vi "UHR-Fleezers Control (fpga) - avogadro 1.vi"() -> ()   [LabVIEW 2014]
doc: "UHR-Fleezers Instrument Control Code (fpga)"
uses:
  <vilib>/Platform/TimedLoop/XDataNode/timing_clust.ctl
  <vilib>/Platform/TimedLoop/XDataNode/nitl_modes.ctl
  <vilib>/Platform/TimedLoop/XDataNode/wakeup.ctl
  <vilib>/rvi/Emulation/niFpgaGetClockAttributes.vi
  <vilib>/rvi/Emulation/niFpgaSctlEmulationGetInTimedLoop.vi
  <vilib>/rvi/Emulation/niFpgaEmulationReportErrorSimple.vi
  <vilib>/rvi/Emulation/niFpgaProcessEmulError.vi
  <vilib>/rvi/eio/common/nirviEmuTemplateMethod_errors.vi
  <vilib>/rvi/interface/RandomDataEmulation/niFpgaRandomDataHandleErrors.vi
  <vilib>/rvi/Emulation/niFpgaCriticalErrorInLSC.vi
  <vilib>/eio/EIONode/EIONode.xnode
  <vilib>/eio/EIOMethodNode/EIOMethodNode.xnode
  <vilib>/rvi/DataTransferAndStorage/Container/XNode/niFpgaContainer.xnode
  <vilib>/rvi/interface/RandomDataEmulation/nirviRandomDataFpgaReadWriteTemplate.vi
  <vilib>/addons/control/pid/fpga.llb/XNode/niFpgaPID.xnode
  <vilib>/Platform/TimedLoop/XDataNode/XDataNode.xnode
  <vilib>/Platform/TimedLoop/XDataNode/XDNodeRunTimeDep.lvlib
panel:
  in  "Tab Control":T1(tab)=enum."MCL trap control"
  in  "Set 3":bool
  in  "Set 2":bool=TRUE
  in  "Set 1":bool=TRUE
  in  "Trap Pos to FIFO":bool
  in  "N of AI1 Int Acq Sets":i16=2 min=1 max=3 step=1
  out "AI Late Counter":u8
  in  "ai count":u16=400
  in  "+ phase":bool
  in  "Phase count adjustment":i16
  out "Relative phase":i16
  in  "AI to FIFO":bool
  out "BD1 Frequency Out 1":u64
  out "BD1 Frequency Out 2":u64
  out "Trap Pos FIFO Timeout":u16
  out "Trap AI FIFO Timeout":u16
  in  "Trap FIFO Set Timeout":i32
  in  "Tab Control 2":T2(tab)
  in  "FB output range":cluster{"output low":i16, "output high":i16}={"output low"=0, "output high"=3000}
  in  "FB Gains":T3={"proportional gain (Kc)"=10, "integral gain (Kc*Ts/Ti)"=5, "derivative gain (Kc*Td/Ts)"=0}
  in  "RD":bool
  in  "Swap F1 and F2":bool
  in  "Cont. Scan":bool
  in  "Abort scan":bool
  in  "Cycles per step":u64
  in  "Scan BD":bool
  in  "Number of scans":u16
  in  "Scan steps":u64
  in  "Scan freq.  increment":i64
  out "Scanning":bool
  in  "Start scan":bool
  in  "OSK Bd 1":bool
  in  "Reset Bd 1":bool
  in  "PMODE":bool
  in  "Direct RF Box \nCommunication":bool
  in  "Data BD 2":u8 format="%08b"
  in  "Data BD 1":u8 format="%08b"
  in  "Address":u8 format="%02x"
  in  "Update Data":bool
  in  "FPGA Controls\n RF Box":bool
  in  "Number Interlace Cycles":u8=2 min=1 max=3
  in  "Interlace Off Parameters":u8=1 min=1 max=3
  in  "Interlace ON/OFF":bool
  out "DIO Relative phase":i16
  in  "Phase count adjustment (DIO)":i16
  in  "+ phase (DIO)":bool
  out "DIO Late Counter":u8
  in  "DIO count 1 (ticks)":u16=400
  in  "DIO count 2 (ticks)":u16=400
  in  "DIO count 3 (ticks)":u16=400
  out "AI2 Y Sum Set 2":i16
  out "AI2 Y Sum Set 1":i16
  in  "FB Setpoint Set 1":i16 min=0 step=1
  in  "FB Reset Set 1":bool
  in  "FB On/Off Set 1":bool
  in  "FB Reset Set 2":bool
  in  "FB On/Off Set 2":bool
  in  "FB Setpoint Set 2":i16 min=0 step=1
  out "Scan I":u64
  in  "Amp switch delay":u8=5
  in  "BD 2 Amplitude 1":u16
  in  "BD 1 Amplitude 1":u16
  in  "BD 2 Frequency 1":u64
  in  "BD 1 Frequency 1":u64
  in  "BD 2 Amplitude 2":u16
  in  "BD 1 Amplitude 2":u16
  in  "BD 2 Frequency 2":u64
  in  "BD 1 Frequency 2":u64
  in  "BD 2 Amplitude 3":u16
  in  "BD 1 Amplitude 3":u16
  in  "BD 2 Frequency 3":u64
  in  "BD 1 Frequency 3":u64
  in  "BD 1 Delay (ticks)":u8
  in  "BD 2 Delay (Ticks)":u8 caption="Count(Ticks)"
  in  "Next trap write delay (ticks)":u8 caption="Count(Ticks)"
  out "Piezo X out":i16
  out "Piezo Y out":i16
  in  "Piezo Trap ON/Off (AO3)":i16
  in  "Piezo Trap X (AO5)":i16
  in  "Piezo Trap Y (AO4)":i16
  in  "Trap pos. FB Range":T4={"FB2 output low"=-1.0, "FB2 output high"=0.999969482421875}
  in  "FB Min frequency":u64
  in  "FB Max Frequency":u64
  in  "Dynamic Force FB (Ronen)":bool
  in  "Negate Diff?":bool
  in  "Diff FB Measurement?":bool
  in  "FB Trig Integrate":u32=1
  out "TTrig?":bool
  in  "TTrig Negate Pos":bool=TRUE
  out "Trap Pos FB Int Signal":fxp<+/-,24,9> format="%.18g"
  out "Trap Pos FB Int-Norm Signal":fxp<+/-,16,1> format="%.16g"
  in  "FPGA TTrig Thresh":i64
  in  "FPGA Trap Trig":bool
  out "Trap Pos FB Action":i64
  in  "Trap Pos. FB Offset Factor":i64
  in  "Trap Pos. FB Mult Factor":i64=2
  in  "Trap Pos. FB Reset":bool
  in  "Trap Pos FB Monitor T1 or T2":bool
  in  "AI1 X Scale":u16
  in  "Trap Pos FB Int Count":u16=100
  in  "Trap Pos FB Negate Action":bool
  out "AI1 X Set 2":fxp<+/-,16,1>
  out "AI1 X Set 1":fxp<+/-,16,1>
  in  "Trap Pos. FB SP":fxp<+/-,16,1>
  in  "Force feedback":bool
  out "TTrig Sig":i64
  out "TTrig Fin Thresh":i64
  in  "B factor":fxp<+/-,32,16>
  in  "Trap Pos. FB Gains":T5={"proportional gain (Kc)"=0.999969482421875, "integral gain (Kc*Ts/Ti)"=0.999969482421875, "derivative gain (Kc*Td/Ts)"=0.0}
  in  "ScanTrap 3 or Fl-laser":bool
  in  "1D or 2D Scan?":bool
  in  "Abort scan (MCL)":bool
  in  "MCL Scan Axis":bool
  in  "Cont. Scan (MCL)":bool
  out "Scan I (MCL)":u64
  in  "Number of scans (MCL)":u16
  out "Scanning MCL":bool
  in  "Scan steps (MCL)":u64
  in  "Cycles per step (MCL)":u64
  in  "Scan freq.  increment (MCL)":i16
  in  "Start scan (MCL)":bool
  in  "AO2 (X)":i16
  in  "AO1 (Y)":i16
  out "MCL Late Counter":u8
  in  "MCL count":u32=800
  out "MCL Relative Phase":i16
  in  "Phase count adjustment (MCL)":i16
  in  "+ phase (MCL)":bool
  out "APD2 int gate":bool
  out "APD3 out state":bool
  in  "APD Gate Operating Mode":u8 max=2 step=1
  in  "Invert APD Gate":bool
  in  "APD Gate OFF Count":u16=100
  in  "APD Gate ON Count":u16=300
  out "APD 1 Gate Late Counter":u8
  out "APD 1 Gate Relative Phase":i16
  in  "Phase count adjustment (APD 1 Gate)":i16
  in  "+ phase (APD 1 Gate)":bool
  out "APD 2 Counts 0":u32
  out "APD 2 Counts 1":u32
  out "APD 1 Counts 0":u32
  out "APD 1 Counts 1":u32
  out "APD1 out state":bool
  in  "APD AO scale factor":i16=1
  in  "APD to FIFO":bool
  in  "APD Acq Rate Count":u32=20000000
  out "APD Acq Late Counter":u8
  out "APD Acq Relative Phase":i16
  in  "Phase Count Adjustment (APD Acq)":i16
  in  "+ phase (APD Acq)":bool
  in  "Phase count adjustment (APD 2 Gate)":i16
  out "APD 2 Gate Late Counter":u8
  out "APD 2 Gate Relative Phase":i16
  in  "+ phase (APD 2 Gate)":bool
  out "APD2 out state":bool
  out "APD 3 Counts 0":u32
  out "APD 3 Counts 1":u32
  out "APD 3 Gate Late Counter":u8
  in  "Phase count adjustment (APD 3 Gate)":i16
  out "APD 3 Gate Relative Phase":i16
  in  "+ phase (APD 3 Gate)":bool
  out "APD1 int gate":bool
  out "APD3 int gate":bool
  in  "D3":i16
  in  "I3":i16=5
  in  "P3":i16=10
  in  "Green Filter Flipper":bool
  in  "Green FB Count":u16=1200
  out "Green Late Counter":u8
  out "Green FB Relative Phase":i16
  in  "Phase count adjustment (Green FB)":i16=10
  in  "+ phase (Green FB)":bool
  out "Green FB Sum":i16
  in  "Green int current ON count adj":u16=150
  in  "Current Out":u16=30000
  in  "Green FB On/Off":bool
  in  "Green FB Setpoint":i16=250 min=0 step=1
  in  "Green FB Reset":bool
  in  "Operating Mode 2":u8=2 max=2 step=1
  in  "Invert GI 2":bool
  in  "Green interlace OFF count 2":u16=900
  in  "Green interlace ON count 2":u16=300
  out "GI Late Counter 2":u8
  out "GI Relative phase 2":i16
  in  "Phase count adjustment (GI) 2":i16=20
  in  "+ phase (GI) 2":bool
  in  "Green interlace OFF count":u16=100
  out "GI Relative phase":i16
  in  "Phase count adjustment (GI)":i16
  in  "+ phase (GI)":bool
  in  "Green interlace ON count":u16=300
  out "GI Late Counter":u8
  in  "Invert GI":bool
  in  "Operating Mode":u8 max=2 step=1
  in  "+ phase (RI)":bool
  out "RI Relative phase":i16
  out "RI Late Counter":u8
  in  "Red interlace ON count":u16=300
  in  "Red interlace OFF count":u16=100
  in  "Invert RI":bool
  in  "Red Laser Operating Mode":u8 max=2 step=1
  in  "Phase count adjustment (RI)":i16
  out "Red FB Intensity":i16
  in  "RI Current Out":u16=30000
  in  "Red FB On/Off":bool
  in  "D4":i16
  in  "I4":i16=5
  in  "P4":i16=10
  in  "Red FB Setpoint":i16=250 min=0 step=1
  in  "Red FB Reset":bool
  in  "RI Operating Mode 2":u8=2 max=2 step=1
  in  "Invert RI 2":bool
  in  "Phase count adjustment (BI AO)":i16=20
  in  "Blue current ON count adj (AO)":u16=150
  in  "BI Current Out":i16=30000
  in  "Blue FB On/Off":bool
  in  "D5":i16
  in  "I5":i16=5
  in  "P5":i16=10
  in  "Blue FB Setpoint":i16=250 min=0 step=1
  in  "Blue FB Reset":bool
  in  "BI Operating Mode (AO)":u8=2 max=2 step=1
  in  "Invert BI (AO)":bool
  in  "Blue OFF count (AO)":u16=900
  in  "Blue ON count (AO)":u16=300
  out "BI Late Counter (AO)":u8
  out "BI Relative phase (AO)":i16
  in  "+ phase (BI AO)":bool
  in  "Phase count adjustment (BI D)":i16
  in  "Blue Laser Operating Mode (D)":u8 max=2 step=1
  in  "Invert BI (D)":bool
  in  "Blue interlace OFF count (D)":u16=100
  in  "Blue interlace ON count (D)":u16=300
  out "Blue Late Counter (D)":u8
  out "BI Relative phase (D)":i16
  in  "+ phase (BI D)":bool
  out "Blue Intensity":i16
  # "Only one of these can be on\nat a time:"
  # "Raster Scan AOD"
  # "1 (X)"
  # "2 (Y)"
  # "IR Intensity Feedback (RF BD 1)"
  # "False is usual, True is external loop method"
  # "Parameters if using the external RF switching loop"
  # "Parameters if using the usual internal RF switching method"
  # "FB Triggering Excitation Laser"
  # "Trap Pos. FB Gains"
  # "Trap Pos. FB Range"
  # "AO1 (Y)"
  # "2D"
  # "Trap 3"
  # "1D"
  # "Fl Laser"
  # "AO2 (X)"
  # "APD AO for aligning"
  # "Detection Loop"
  # "Green fluorescent laser digital gate interlacing loop"
  # "0 Forced ON\n1 Forced OFF\n2 Interlacing"
  # "Green FB Gains"
  # "Red fluorescent laser digital gate interlacing loop"
  # "Detection Loop"
  # "0 Forced ON\n1 Forced OFF\n2 Interlacing"
  # "Analog/FB Control Loop\n(Disabled)"
  # "Digital Control Loop"
  # "Blue laser intensity reading"
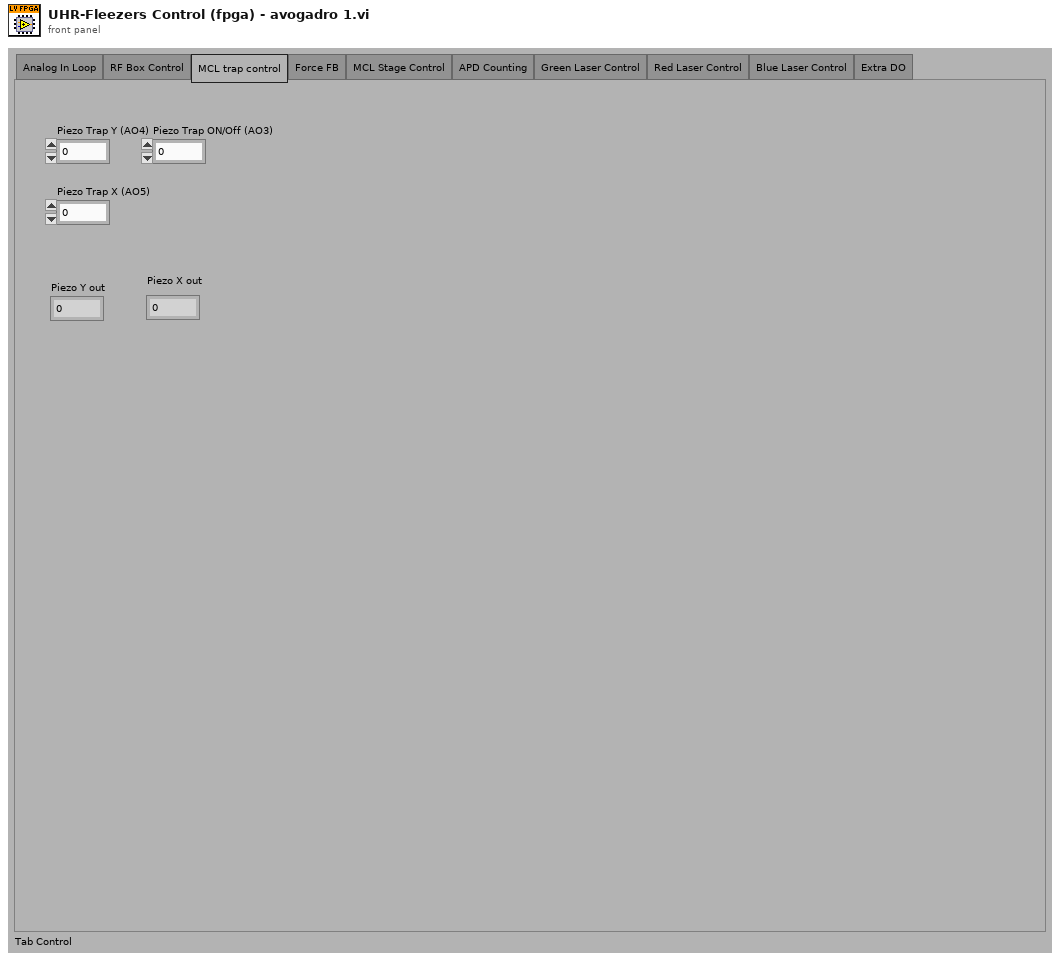
[diagram p1: front panel]
types:
  T1 = enum32{"Analog In Loop", "RF Box Control", "MCL trap control", "Force FB", "MCL Stage Control", "APD Counting", "Green Laser Control", "Red Laser Control", "Blue Laser Control", "Extra DO"}
  T2 = enum32{"Controls", "Interlacing Frequency and Amplitude Values", "Oscillate trap from memory"}
  T3 = cluster{"proportional gain (Kc)":i16, "integral gain (Kc*Ts/Ti)":i16, "derivative gain (Kc*Td/Ts)":i16}
  T4 = cluster{"FB2 output low":fxp<+/-,16,1>, "FB2 output high":fxp<+/-,16,1>}
  T5 = cluster{"proportional gain (Kc)":fxp<+/-,16,1>, "integral gain (Kc*Ts/Ti)":fxp<+/-,16,1>, "derivative gain (Kc*Td/Ts)":fxp<+/-,16,1>}
  T6 = typedef "XDNodeRunTimeDep.lvlib/timing_clust.ctl" = cluster{"Expected End [f-1]":u64, "Actual End [f-1]":u64, "Finished Late? [f-1]":bool, "Expected End [i-1]":u64, "Actual End [i-1]":u64, "Finished Late? [i-1]":bool, "Expected Start [i]":u64, "Actual Start [i]":u64, "Expected Start [f]":u64, "Actual Start [f]":u64, "Source Name":string, "Structure Name":string, "Period":i64, "Deadline":i64, "Offset":i64, "Start":i64, "Priority":i32, "Timeout":i32, "Mode":T7, "Wakeup Reason":T8, "Error":errorcluster, "Source Type":string, "Secondary Source Type":string, "Global End Time":u64, "Global Start Time":u64, "Frame Duration":u64, "Iteration Duration":u64, "Assigned CPU":i32, "I/O Scan Engine Mode":u32}
  T7 = typedef "XDNodeRunTimeDep.lvlib/nitl_modes.ctl" = enum32{"No Change", "Process missed periods, maintain original phase", "Discard missed periods, maintain original phase", "Process missed periods, ignore original phase", "Discard missed periods, ignore original phase"}
  T8 = typedef "XDNodeRunTimeDep.lvlib/wakeup.ctl" = enum32{"Normal", "Aborted", "Asynchronous wakeup", "Timing source error", "Timed loop error", "Timeout"}
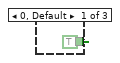
[diagram p2: hidden frame]
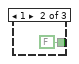
[diagram p3: hidden frame]
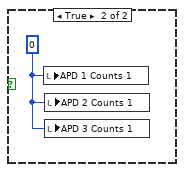
[diagram p5: hidden frame]
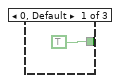
[diagram p7: hidden frame]
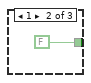
[diagram p8: hidden frame]
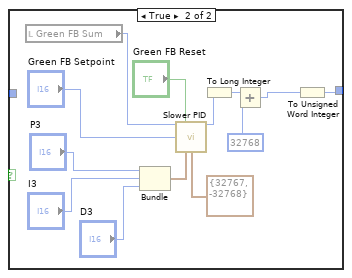
[diagram p11: hidden frame]
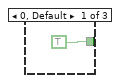
[diagram p12: hidden frame]
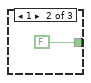
[diagram p13: hidden frame]
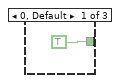
[diagram p14: hidden frame]
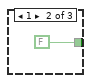
[diagram p15: hidden frame]
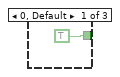
[diagram p17: hidden frame]
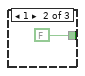
[diagram p18: hidden frame]
diagram:
  w1 = i16 0
  w6 = FALSE
  w4 = FALSE
  # "Control of MCL trap"
  # "timing array current index"
  # "timing array"
  # "timing counter (phase adjusted here)"
  # "late counter"
  n1 = flat-sequence "FPGA initialization to do before running any of the loops" {
    tunnel: [u16 0 ("DIO count 3 (ticks)")] -> w2
    tunnel: [w14] -> _
    frame #0 {
      w13 = FALSE ("Enable")
      # "BD 2 (Y)"
      # "BD 1 (X)"
      # "Start up expansion chassis early\nto avoid delays later"
      # "This pin controls udclk on the RF boards.\nWhen initially configuring the boards, this pin needs to be\nconfigured as a high impedance input.  Later it will be switched\nto an output."
      # "Initial setting of DIO data and \naddress to low (before reset).  \nThis needs to happen before the other\ncontrol method loops execute."
      n2 = xnode "FPGA I/O Node"("Chassis2/Mod1/AO0"=u16 0 ("Chassis2/Mod4/AO0")) -> ("Chassis2/Mod2/AI0"=w14:i16)  [unwired: 2 in, 2 out]
      n3 = xnode "FPGA I/O Method Node"("Enable"=w13) -> ()  [unwired: 1 in, 1 out]
      n4 = xnode "FPGA I/O Method Node"("Enable"=w13) -> ()  [unwired: 1 in, 1 out]
      n5 = xnode "FPGA I/O Node"("Connector1/DIO0"=FALSE, "Connector1/DIO1"=FALSE, "Connector1/DIO2"=FALSE, "Connector1/DIO3"=FALSE, "Connector1/DIO4"=FALSE, "Connector1/DIO5"=FALSE, "Connector1/DIO6"=FALSE, "Connector1/DIO7"=FALSE, "Connector1/DIO8"=FALSE, "Connector1/DIO9"=FALSE, "Connector1/DIO10"=FALSE, "Connector1/DIO11"=FALSE, "Connector1/DIO12"=FALSE, "Connector1/DIO13"=FALSE, "Connector1/DIO15"=FALSE, "Connector1/DIO20"=FALSE, "Connector1/DIO21"=FALSE, "Connector1/DIO22"=FALSE, "Connector1/DIO23"=FALSE, "Connector1/DIO24"=FALSE, "Connector1/DIO25"=FALSE, "Connector1/DIO26"=FALSE, "Connector1/DIO27"=FALSE, "Connector1/DIO14"=FALSE) -> ()  [unwired: 24 in, 24 out]
    }
  }
  n6 = local read "AO1 (Y)"() -> (w11:i16)
  n7 = local read "AO2 (X)"() -> (w10:i16)
  n8 = node-c288() -> (w9:T6)  [unwired: 1 in]
  n9 = To Unsigned Long Integer(number=w2) -> (unsigned 32bit integer=w7:u32)
  n10 = timed-loop "RF box board DIO control: control bits" {
    timing: w9 -> [_]
    timing-out: [_] -> w8
    tunnel: [w43] -> _
    tunnel: w2 -> [w43]
    stop <- FALSE stop-if-true
    n11 = xnode "FPGA I/O Node"("Connector1/DIO16"="RD", "Connector1/DIO17"="PMODE", "Connector1/DIO18"="OSK Bd 1", "Connector1/DIO19"="Reset Bd 1", "Connector0/DIO3"="Green Filter Flipper") -> ()  [unwired: 5 in, 5 out]
  }
  n12 = while "RF box board DIO control: parallel communication" {
    shift-right: [w58] -> _
    shift-left: w2 -> [w57]
    shift-right: [w56] -> _
    shift-left: FALSE ("Swap F1 and F2") -> [w55]
    shift-right: [w50] -> _
    shift-left: u64 0 -> [w51]
    stop <- FALSE stop-if-true
    n13 = flat-sequence {
      tunnel: w55 -> [w62]
      tunnel: w57 -> [w60]
      tunnel: [w62] -> w54
      tunnel: [w61] -> w53
      tunnel: [w60] -> w52
      tunnel: [w70] -> w58
      tunnel: [w69] -> w56
      tunnel: w54 -> [w68]
      tunnel: w53 -> [w66]
      tunnel: w52 -> [w65]
      tunnel: w51 -> [w64]
      tunnel: [w63] -> w50
      frame #0 {
        n14 = call "Loop Timer"("Count(Ticks)"=w60) -> ("Tick Count(Ticks)"=w61:u16)
      }
      frame #1 {
        n15 = flat-sequence {
          tunnel: ["FPGA Controls\n RF Box"] -> w67
          tunnel: w68 -> [w71]
          tunnel: [w123] -> w70
          tunnel: [w136] -> w69
          tunnel: w67 -> [w135]
          tunnel: w66 -> [w129]
          tunnel: w65 -> [w126]
          tunnel: w64 -> [w101]
          tunnel: [w100] -> w63
          frame #0 {
            n16 = case shown="True" "FPGA Controls\n RF Box" {
              tunnel: w71 -> [_ w73]
              frame False {
              }
              frame True {
                n17 = flat-sequence {
                  tunnel: w73 -> [w83]
                  frame #0 {
                    n18 = First Call?() -> (First Call?: T/F=w74:bool)
                    n19 = case shown="True" w74 {
                      frame False {
                      }
                      frame True {
                        # "BD 2"
                        # "BD 1"
                        # "If first time data updated, be sure to set WR high and UDCLK low\nbefore setting data and address bits."
                        n20 = xnode "FPGA I/O Method Node"("Enable"=TRUE) -> ("FPGA I/O Out"=w76:refnum<k21>)  [unwired: 1 in]
                        n21 = xnode "FPGA I/O Method Node"("Enable"=TRUE) -> ("FPGA I/O Out"=w79:refnum<k21>)  [unwired: 1 in]
                        n22 = xnode "FPGA I/O Node"("Connector1/DIO15"=TRUE) -> ()  [unwired: 1 in, 1 out]
                        n23 = xnode "FPGA I/O Node"("I/O Item"=FALSE ("Connector1/DIO30"), "FPGA I/O In"=w76) -> ()  [unwired: 1 out]
                        n24 = xnode "FPGA I/O Node"("I/O Item"=FALSE ("Connector1/DIO30"), "FPGA I/O In"=w79) -> ()  [unwired: 1 out]
                      }
                    }
                  }
                  frame #1 {
                    n25 = case shown="False" FALSE {
                      tunnel: w83 -> [w85 _]
                      frame False {
                        # "Usual operation"
                        n26 = disable-structure shown="Disabled" {
                          disable-tunnel: w85 -> [w87 _]
                          disable-tunnel: "Amp switch delay" -> [w86 _]
                          frame Disabled {
                            n27 = flat-sequence "BD 2 (Y)" {
                              tunnel: w87 -> [w89]
                              tunnel: w86 -> [w90]
                              frame #0 {
                                n28 = call "Wait7"("Count(Ticks)"="BD 2 Delay (Ticks)") -> ()  [unwired: 1 out]
                              }
                              frame #1 {
                                # "switch frequency"
                                n29 = xnode "FPGA I/O Node"("Connector1/DIO37"=w89) -> ()  [unwired: 1 in, 1 out]
                              }
                              frame #2 {
                                # "~5 ticks is usual"
                                n30 = call "Wait5"("Count(Ticks)"=w90) -> ()  [unwired: 1 out]
                              }
                              frame #3 {
                                # "this switches amplitude"
                                # "switch amplitude"
                                # "send udclk high"
                                n31 = xnode "FPGA I/O Node"("Connector1/DIO29"=TRUE ("Connector1/DIO15")) -> ()  [unwired: 1 in, 1 out]
                              }
                              frame #4 {
                                # "reset to be ready for next\ncycle"
                                # "send udclk low"
                                n32 = xnode "FPGA I/O Node"("Connector1/DIO29"=FALSE ("Connector1/DIO15")) -> ()  [unwired: 1 in, 1 out]
                              }
                            }
                          }
                          frame Enabled {
                          }
                        }
                        n33 = flat-sequence "BD 1 (X)" {
                          tunnel: w85 -> [w94]
                          tunnel: "Amp switch delay" -> [w95]
                          frame #0 {
                            n34 = call "Wait6"("Count(Ticks)"="BD 1 Delay (ticks)") -> ()  [unwired: 1 out]
                          }
                          frame #1 {
                            # "switch frequency"
                            n35 = xnode "FPGA I/O Node"("Connector1/DIO36"=w94) -> ()  [unwired: 1 in, 1 out]
                          }
                          frame #2 {
                            # "~5 ticks is usual"
                            n36 = call "Wait4"("Count(Ticks)"=w95) -> ()  [unwired: 1 out]
                          }
                          frame #3 {
                            # "this switches amplitude"
                            # "switch amplitude"
                            # "send udclk high"
                            n37 = xnode "FPGA I/O Node"("Connector1/DIO30"=TRUE ("Connector1/DIO15")) -> ()  [unwired: 1 in, 1 out]
                          }
                          frame #4 {
                            # "reset to be ready for next\ncycle"
                            # "send udclk low"
                            n38 = xnode "FPGA I/O Node"("Connector1/DIO30"=FALSE ("Connector1/DIO15")) -> ()  [unwired: 1 in, 1 out]
                          }
                        }
                      }
                      frame True {
                        # "Operation when you need a long delay for either X or Y to synchonize AOD light out phase (> ~100 ticks)."
                        # "Trigger the external loop by sending the boolean FSK value through a FIFO"
                      }
                    }
                  }
                  frame #2 {
                  }
                }
              }
            }
          }
          frame #1 {
            # "This is the prior cycle's on time"
            # "increment timing\nindex, reset to 0 if \nend of matrix"
            # "Reset to begginning (1) when number of cycles reached."
            # "timing index"
            # "build byte stacks for writing data\n(must correspond to addresses array constant)"
            # "Timing housekeeping"
            # "Adjust phase if late\n(maintains constant phase relationship between cycles)"
            n39 = feedback #1(u8 0 ("t")) -> (w132:u8)
            n40 = Increment(x=w132) -> (x+1=w175:u8)
            n41 = Increment(x="Number Interlace Cycles") -> (x+1=w170:u8)
            n42 = Equal?(x=w175, y=w170) -> (x = y?=w177:bool)
            n43 = Select(t=u8 1, s=w177, f=w175) -> (s? t:f=w131:u8)
            n44 = feedback-in #1(w131) -> ()
            n45 = Increment(x=w131) -> (x+1=w172:u8)
            n46 = Equal?(x=w172, y=w170) -> (x = y?=w173:bool)
            n47 = Select(t=u8 1, s=w173, f=w172) -> (s? t:f=w169:u8)
            n48 = Select(t=w169, s="Interlace ON/OFF", f="Interlace Off Parameters") -> (s? t:f=w102:u8)
            n49 = case shown="1, Default" w102 {
              tunnel: [w221 w430 "BD 1 Frequency 3"] -> w165
              tunnel: [w264 "BD 2 Frequency 2" "BD 2 Frequency 3"] -> w154
              tunnel: ["BD 2 Amplitude 1" "BD 2 Amplitude 2" "BD 2 Amplitude 3"] -> w111
              tunnel: [w230 w428 "BD 1 Amplitude 3"] -> w114
              tunnel: "FB output range" -> [w234 w425 _]
              tunnel: w101 -> [w229 w427 w443]
              tunnel: [w221 w427 w443] -> w100
              tunnel: "FB Gains" -> [w216 w426 _]
              frame 1, Default {
                w248 = fxp<+/-,24,9> 0.0 ("AI1 X Set 2")
                w242 = u16 0
                w260 = u64 0 ("f")
                # "Added by Ronen -\nUpper and Lower \nLimits for the FB \ngenerated frequency\nto avoid losing bead \nwhen tether breaks"
                # "Changed by Ronen - correction \nby PID is now implemented not on \nthe Base BD1 frequency but on the last\nfrequency sent."
                # "BD1 Amp 1"
                # "This signal integration happens no matter what\nso that correct setpoints can be chosen before \nturning on the FB."
                # "Trap 1"
                n50 = local read "AI1 X Set 2"() -> (w224:fxp<+/-,16,1>)
                n51 = local read "AI1 X Set 1"() -> (w245:fxp<+/-,16,1>)
                n52 = local read "Scanning"() -> (w265:bool)
                n53 = Multiply(x=w224, y="B factor") -> (x*y=w222:fxp<+/-,48,17>)
                n54 = Or(x=w265, y="Start scan") -> (x .or. y?=w258:bool)
                n55 = case shown="True" "Diff FB Measurement?" {
                  tunnel: w222 -> [w283 w292]
                  tunnel: w245 -> [w282 w293]
                  tunnel: [w280 w284] -> w246
                  frame False {
                    n56 = Select(t=w282, s="Trap Pos FB Monitor T1 or T2", f=w283) -> (s? t:f=w280:fxp<+/-,48,17>)
                  }
                  frame True {
                    n57 = Subtract(x=w293, y=w292) -> (x-y=w285:fxp<+/-,48,17>)
                    n58 = Not(x="Negate Diff?") -> (.not. x?=w291:bool)
                    n59 = Boolean To (0,1)(Boolean="Negate Diff?") -> (0, 1=w289:i16)
                    n60 = Boolean To (0,1)(Boolean=w291) -> (0, 1=w290:i16)
                    n61 = Negate(x=w289) -> (-x=w288:i16)
                    n62 = Add(x=w288, y=w290) -> (x+y=w286:i16)
                    n63 = Multiply(x=w286, y=w285) -> (x*y=w284:fxp<+/-,63,32>)
                  }
                }
                n64 = Not(x="Abort scan") -> (.not. x?=w256:bool)
                n65 = And(x=w256, y=w258) -> (x .and. y?=w255:bool)
                n66 = case "For raster scanning" shown="True" w255 {
                  tunnel: [u64 0 w415] -> w261
                  tunnel: "Start scan" -> [_ w400]
                  frame False {
                    n67 = local write "Scanning"(FALSE ("scanning")) -> ()
                  }
                  frame True {
                    w384 = i64 0
                    w383 = u64 0
                    # "scan incr."
                    # "freq. incr. mult."
                    # "count steps"
                    # "count number of cycles"
                    n68 = feedback #2(w383) -> (w412:u64)
                    n69 = Select(t=w383, s=w400, f=w412) -> (s? t:f=w414:u64)
                    n70 = Increment(x=w414) -> (x+1=w411:u64)
                    n71 = Greater?(x="Cycles per step", y=w411) -> (0:w393:bool)
                    n72 = Select(t=w411, s=w393, f=w383) -> (s? t:f=w410:u64)
                    n73 = feedback-in #2(w410) -> ()
                    n74 = feedback #3(w383) -> (w409:u64)
                    n75 = Select(t=w383, s=w400, f=w409) -> (s? t:f=w404:u64)
                    n76 = Increment(x=w404) -> (x+1=w408:u64)
                    n77 = Add(x="Scan steps", y="Scan steps") -> (x+y=w407:u64)
                    n78 = Select(t=w404, s=w393, f=w408) -> (s? t:f=w388:u64)
                    n79 = Greater?(x=w407, y=w388) -> (0:w387:bool)
                    n80 = Select(t=w388, s=w387, f=w383) -> (s? t:f=w405:u64)
                    n81 = feedback-in #3(w405) -> ()
                    n82 = Equal?(x="Scan steps", y=w388) -> (x = y?=w392:bool)
                    n83 = Greater?(x="Scan steps", y=w404) -> (0:w403:bool)
                    n84 = feedback #4(w384) -> (w406:i64)
                    n85 = Select(t=w384, s=w400, f=w406) -> (s? t:f=w390:i64)
                    n86 = Increment(x=w390) -> (x+1=w402:i64)
                    n87 = Decrement(x=w390) -> (x-1=w401:i64)
                    n88 = Select(t=w402, s=w403, f=w401) -> (s? t:f=w391:i64)
                    n89 = Select(t=w390, s=w392, f=w391) -> (s? t:f=w389:i64)
                    n90 = Select(t=w390, s=w393, f=w389) -> (s? t:f=w385:i64)
                    n91 = Select(t=w385, s=w387, f=w384) -> (s? t:f=w386:i64)
                    n92 = feedback-in #4(w386) -> ()
                    n93 = feedback #5(w383) -> (w399:u64)
                    n94 = Select(t=w383, s=w400, f=w399) -> (s? t:f=w395:u64)
                    n95 = Increment(x=w395) -> (x+1=w396:u64)
                    n96 = Select(t=w395, s=w387, f=w396) -> (s? t:f=w394:u64)
                    n97 = Greater?(x="Number of scans", y=w394) -> (0:w380:bool)
                    n98 = Multiply(x="Scan freq.  increment", y=w390) -> (x*y=w415:i64)
                    n99 = Select(t=TRUE, s="Cont. Scan", f=w380) -> (s? t:f=w379:bool)
                    "Scanning" <- w379
                    n100 = Select(t=w394, s=w379, f=w383) -> (s? t:f=w397:u64)
                    n101 = feedback-in #5(w397) -> ()
                    n102 = Increment(x=w394) -> (x+1=→"Scan I":u64)
                  }
                }
                n103 = feedback #6(w242) -> (w241:u16)
                n104 = Increment(x=w241) -> (x+1=w243:u16)
                n105 = Greater Or Equal?(x=w243, y="Trap Pos FB Int Count") -> (x >= y?=w228:bool)
                n106 = Select(t=w242, s=w228, f=w243) -> (s? t:f=w244:u16)
                n107 = feedback-in #6(w244) -> ()
                n108 = feedback #7(w248) -> (w247:fxp<+/-,24,9>)
                n109 = Add(x=w246, y=w247) -> (x+y=w240:fxp<+/-,24,9>)
                n110 = case "For intensity feedback" shown="True" "FB On/Off Set 1" {
                  tunnel: [w417 w423] -> w230
                  tunnel: w234 -> [_ w424]
                  tunnel: "BD 1 Amplitude 1" -> [w417 _]
                  tunnel: w216 -> [_ w418]
                  frame False {
                  }
                  frame True {
                    n111 = local read "AI2 Y Sum Set 1"() -> (w421:i16)
                    n112 = call "Slower PID.vi"("process variable"=w421, "reset?"="FB Reset Set 1", "setpoint"="FB Setpoint Set 1", "PID gains (x 2^8)"=w418, "output range"=w424) -> ("output"=w419:i16)  [unwired: 10 out]
                    n113 = To Unsigned Word Integer(number=w419) -> (unsigned 16bit integer=w423:u16)
                  }
                }
                n114 = Select(t=w248, s=w228, f=w240) -> (s? t:f=w251:fxp<+/-,24,9>)
                n115 = feedback-in #7(w251) -> ()
                n116 = Divide(x=w240, y="Trap Pos FB Int Count") -> (x/y=w235:fxp<+/-,16,1>)
                n117 = feedback #8(fxp<+/-,24,9> 0.0 ("AI1 X Set 2")) -> (w252:fxp<+/-,24,9>)
                n118 = Select(t=w240, s=w228, f=w252) -> (s? t:f=w253:fxp<+/-,24,9>)
                "Trap Pos FB Int Signal" <- w253
                n119 = feedback-in #8(w253) -> ()
                n120 = feedback #9(fxp<+/-,16,1> 0.0 ("Trap Pos FB Int-Norm Signal")) -> (w237:fxp<+/-,16,1>)
                n121 = Select(t=w235, s=w228, f=w237) -> (s? t:f=w236:fxp<+/-,16,1>)
                "Trap Pos FB Int-Norm Signal" <- w236
                n122 = feedback-in #9(w236) -> ()
                n123 = case "For position feedback" shown="True" "Force feedback" {
                  tunnel: [i64 0 w299] -> w233
                  tunnel: w235 -> [_ w296]
                  tunnel: w228 -> [_ w295]
                  frame False {
                  }
                  frame True {
                    n124 = feedback #10(i64 0) -> (w298:i64)
                    n125 = case shown="True" w295 {
                      tunnel: [w300 w304] -> w299
                      tunnel: w298 -> [w300 _]
                      tunnel: w296 -> [_ w303]
                      frame False {
                      }
                      frame True {
                        n126 = xnode ("PID")("process variable"=w303, "reset?"="Trap Pos. FB Reset", "setpoint"="Trap Pos. FB SP", "PID gains"="Trap Pos. FB Gains", "output range"="Trap pos. FB Range") -> ("output"=w313:fxp<+/-,16,1>)
                        n127 = Negate(x=w313) -> (-x=w312:fxp<+/-,17,2>)
                        n128 = Select(t=w312, s="Trap Pos FB Negate Action", f=w313) -> (s? t:f=w309:fxp<+/-,17,2>)
                        n129 = Scale By Power Of 2(n=u32 15, x=u32 1) -> (x*2^n=w306:u32)
                        n130 = Multiply(x=w309, y=w306) -> (x*y=w305:fxp<+/-,17,17>)
                        n131 = To Quad Integer(1:w305) -> (0:w317:i64)
                        "Trap Pos FB Action" <- w317
                        n132 = Multiply(x=w317, y="Trap Pos. FB Mult Factor") -> (x*y=w315:i64)
                        n133 = Add(x=w315, y="Trap Pos. FB Offset Factor") -> (x+y=w304:i64)
                        n134 = disable-structure shown="Disabled" {
                          disable-tunnel: w304 -> [w324 _]
                          frame Disabled {
                            w328 = u32 0
                            n135 = feedback #11() -> (w325:i64)  [unwired: 1 in]
                            n136 = Add(x=w324, y=w325) -> (x+y=w322:i64)
                            n137 = feedback #12(w328) -> (w330:u32)
                            n138 = Increment(x=w330) -> (x+1=w319:u32)
                            n139 = Greater Or Equal?(x=w319, y="FB Trig Integrate") -> (x >= y?=w320:bool)
                            n140 = Select(t=i64 0, s=w320, f=w322) -> (s? t:f=w326:i64)
                            n141 = feedback-in #11(w326) -> ()
                            n142 = Select(t=w328, s=w320, f=w319) -> (s? t:f=w329:u32)
                            n143 = feedback-in #12(w329) -> ()
                            n144 = And(x=w320, y="FPGA Trap Trig") -> (x .and. y?=w327:bool)
                            n145 = case "Trap FB trigger excitation laser ON" shown="True" w327 {
                              tunnel: w322 -> [_ w334]
                              tunnel: w319 -> [_ w332]
                              frame False {
                              }
                              frame True {
                                n146 = Not(x="TTrig Negate Pos") -> (.not. x?=w341:bool)
                                n147 = Boolean To (0,1)(Boolean="TTrig Negate Pos") -> (0, 1=w339:i16)
                                n148 = Boolean To (0,1)(Boolean=w341) -> (0, 1=w340:i16)
                                n149 = Negate(x=w339) -> (-x=w338:i16)
                                n150 = Add(x=w338, y=w340) -> (x+y=w337:i16)
                                n151 = Multiply(x=w337, y=w334) -> (x*y=w336:i64)
                                "TTrig Sig" <- w336
                                n152 = Multiply(x="FPGA TTrig Thresh", y=w332) -> (x*y=w333:i64)
                                "TTrig Fin Thresh" <- w333
                                n153 = Greater Or Equal?(x=w336, y=w333) -> (x >= y?=w335:bool)
                                n154 = case shown="True" w335 {
                                frame False {
                                }
                                frame True {
                                w344 = TRUE ("Green FB On/Off")
                                w346 = u8 2 ("Operating Mode")
                                n155 = local write "Operating Mode 2"(w346) -> ()
                                n156 = local write "Operating Mode"(w346) -> ()
                                n157 = local write "Green FB On/Off"(w344) -> ()
                                n158 = local write "FPGA Trap Trig"(FALSE ("FPGA Trap Trig")) -> ()
                                "TTrig?" <- w344
                                }
                                }
                              }
                            }
                          }
                          frame Enabled {
                          }
                        }
                      }
                    }
                    n159 = feedback-in #10(w299) -> ()
                  }
                }
                n160 = And(x="Force feedback", y="Dynamic Force FB (Ronen)") -> (x .and. y?=w218:bool)
                n161 = case shown="True" w218 {
                  tunnel: w233 -> [w271 w275]
                  tunnel: [w270 w274] -> w231
                  tunnel: w229 -> [_ w273]
                  tunnel: w228 -> [_ w272]
                  frame False {
                    # "(BD1 Frequency 1)"
                    n162 = Add(x="BD 1 Frequency 1", y=w271) -> (x+y=w270:u64)
                  }
                  frame True {
                    n163 = case shown="True" w272 {
                      tunnel: w275 -> [_ w279]
                      tunnel: [w276 w278] -> w274
                      tunnel: w273 -> [w276 w277]
                      frame False {
                      }
                      frame True {
                        n164 = Add(x=w277, y=w279) -> (x+y=w278:u64)
                      }
                    }
                  }
                }
                n165 = Select(t=w260, s="Scan BD", f=w261) -> (s? t:f=w259:u64)
                n166 = Select(t=w261, s="Scan BD", f=w260) -> (s? t:f=w262:u64)
                n167 = Add(x=w259, y="BD 2 Frequency 1") -> (x+y=w264:u64)
                n168 = Compound Arithmetic op=ADD(i64 0 ("f"), w231, w262) -> (w227:u64)
                n169 = In Range and Coerce(upper limit="FB Max Frequency", x=w227, lower limit="FB Min frequency") -> (coerced(x)=w221:u64)  [unwired: 1 out]
                "BD1 Frequency Out 1" <- w221
              }
              frame 2 {
                # "Trap 2"
                n170 = case shown="True" "FB On/Off Set 2" {
                  tunnel: ["BD 1 Amplitude 2" w438] -> w428
                  tunnel: w425 -> [_ w439]
                  tunnel: w426 -> [_ w436]
                  frame False {
                  }
                  frame True {
                    n171 = local read "AI2 Y Sum Set 2"() -> (w441:i16)
                    n172 = call "Slower PID.vi"("process variable"=w441, "reset?"="FB Reset Set 2", "setpoint"="FB Setpoint Set 2", "PID gains (x 2^8)"=w436, "output range"=w439) -> ("output"=w437:i16)  [unwired: 10 out]
                    n173 = To Unsigned Word Integer(number=w437) -> (unsigned 16bit integer=w438:u16)
                  }
                }
                n174 = Add(x="BD 1 Frequency 2", y=i64 0 ("f")) -> (x+y=w430:u64)
                "BD1 Frequency Out 2" <- w430
              }
              frame 3 {
                # "Fluorescence period"
              }
            }
            n175 = feedback-in #13(w129) -> ()
            n176 = feedback #13(w129) -> (w128:u16)
            n177 = Select(t=w131, s="Interlace ON/OFF", f="Interlace Off Parameters") -> (s? t:f=w168:u8)
            n178 = Subtract(x=w129, y=w128) -> (x-y=w127:u16)
            n179 = Subtract "The error"(x=w127, y=w126) -> (x-y=w104:u16)
            n180 = case shown="1, Default" w168 {
              tunnel: ["DIO count 1 (ticks)" "DIO count 2 (ticks)" "DIO count 3 (ticks)"] -> w125
              frame 1, Default {
              }
              frame 2 {
              }
              frame 3 {
              }
            }
            n181 = Number To Boolean Array(number=w104) -> (Boolean array=w105:bool[])
            n182 = Or Array Elements(Boolean array=w105) -> (logical OR=w103:bool)
            n183 = Boolean To (0,1)(Boolean=w103) -> (0, 1=w110:i16)
            n184 = To Unsigned Byte Integer(number=w110) -> (unsigned 8bit integer=w107:u8)
            n185 = feedback #14(u8 0) -> (w108:u8)
            n186 = Add(x=w107, y=w108) -> (x+y=w106:u8)
            "DIO Late Counter" <- w106
            n187 = feedback-in #14(w106) -> ()
            n188 = Subtract(x=w125, y=w104) -> (x-y=w124:u16)
            n189 = Split Number(x=w165) -> (hi(x)=w164:u32, lo(x)=w163:u32)
            n190 = Split Number(x=w154) -> (hi(x)=w159:u32, lo(x)=w158:u32)
            n191 = Boolean To (0,1)(Boolean="+ phase (DIO)") -> (0, 1=w121:i16)
            n192 = Split Number(x=w164) -> (lo(x)=w162:u16)  [unwired: 1 out]
            n193 = Split Number(x=w163) -> (hi(x)=w161:u16, lo(x)=w160:u16)
            n194 = Split Number(x=w159) -> (lo(x)=w157:u16)  [unwired: 1 out]
            n195 = Split Number(x=w158) -> (hi(x)=w156:u16, lo(x)=w155:u16)
            n196 = Split Number(x=w114) -> (hi(x)=w116:u8, lo(x)=w115:u8)
            n197 = Split Number(x=w111) -> (hi(x)=w113:u8, lo(x)=w112:u8)
            n198 = Split Number(x=w162) -> (hi(x)=w153:u8, lo(x)=w152:u8)
            n199 = Split Number(x=w161) -> (hi(x)=w151:u8, lo(x)=w150:u8)
            n200 = Split Number(x=w157) -> (hi(x)=w146:u8, lo(x)=w145:u8)
            n201 = Split Number(x=w160) -> (hi(x)=w149:u8, lo(x)=w148:u8)
            n202 = Split Number(x=w156) -> (hi(x)=w144:u8, lo(x)=w143:u8)
            n203 = Split Number(x=w155) -> (hi(x)=w142:u8, lo(x)=w141:u8)
            n204 = Multiply(x=w121, y="Phase count adjustment (DIO)") -> (x*y=w117:i16)
            n205 = feedback #15(i16 0) -> (w119:i16)
            n206 = Subtract(x=w119, y=w117) -> (x-y=w118:i16)
            "DIO Relative phase" <- w118
            n207 = feedback-in #15(w118) -> ()
            n208 = Add(x=w124, y=w117) -> (x+y=w123:u16)
            n209 = Build Array "BD 1 A Stack"(w116, w115) -> (w138:u8[])
            n210 = Build Array "BD 2 A Stack"(w113, w112) -> (w137:u8[])
            n211 = Build Array "BD 1 nu Stack"(w153, w152, w151, w150, w149, w148) -> (w147:u8[])
            n212 = Build Array "BD 2 nu Stack"(w146, w145, w144, w143, w142, w141) -> (w140:u8[])
            n213 = case shown="2" w102 {
              tunnel: [w208 w211] -> w136
              tunnel: [u8 10 u8 4] -> w139
              tunnel: "Swap F1 and F2" -> [w209 w211]
              frame 2 {
                # "F2"
                n214 = Not(x=w209) -> (.not. x?=w208:bool)
              }
              frame 1, Default {
                # "low chooses F1"
                # "F1"
              }
            }
            n215 = case "If FPGA is controlling (toggling) RF synth" shown="True" w135 {
              tunnel: w147 -> [_ w184]
              tunnel: w140 -> [_ w183]
              tunnel: w139 -> [_ w182]
              tunnel: w138 -> [_ w181]
              tunnel: w137 -> [_ w180]
              frame False {
              }
              frame True {
                # "Write next amp.\n(wait until beginning of next loop iteration to update)"
                n216 = flat-sequence "Update the next F1 and F2 frequency value (the actual frequency won't change until FSK is switched).\nThen load the next amplitude value into buffer, but don't update it until the next cycle." {
                  tunnel: w183 -> [w186]
                  tunnel: w184 -> [w187]
                  tunnel: [w187] -> w179
                  tunnel: [w186] -> w178
                  tunnel: w182 -> [w188]
                  tunnel: w179 -> [w190]
                  tunnel: w178 -> [w189]
                  tunnel: w181 -> [w201]
                  tunnel: w180 -> [w200]
                  frame #0 {
                    # "To possibly send\nthese writes to very\nend of loop (for x and\ny phase adjust)"
                    n217 = call "Wait8"("Count(Ticks)"="Next trap write delay (ticks)") -> ()  [unwired: 1 out]
                  }
                  frame #1 {
                    n218 = for {
                      tunnel: w190 -> [w196] mode=indexing
                      tunnel: w189 -> [w195] mode=indexing
                      tunnel: w188 -> [w193]
                      i -> [w194]
                      # "Write next freq."
                      n219 = To Unsigned Byte Integer(number=w194) -> (unsigned 8bit integer=w191:u8)
                      n220 = Add(x=w193, y=w191) -> (x+y=w192:u8)
                      n221 = call "write to RF synth bd.vi"("Address Byte"=w192, "BD 2 Byte"=w195, "BD 1 Byte"=w196) -> ()
                    }
                  }
                  frame #2 {
                    w197 = TRUE ("Connector1/DIO15")
                    # "send udclk high\n(BD 1 and 2)"
                    n222 = xnode "FPGA I/O Node"("Connector1/DIO30"=w197, "Connector1/DIO29"=w197) -> ()  [unwired: 2 in, 2 out]
                  }
                  frame #3 {
                    w198 = FALSE ("Connector1/DIO15")
                    n223 = xnode "FPGA I/O Node"("Connector1/DIO30"=w198, "Connector1/DIO29"=w198) -> ()  [unwired: 2 in, 2 out]
                  }
                  frame #4 {
                    n224 = for {
                      tunnel: w201 -> [w207] mode=indexing
                      tunnel: w200 -> [w206] mode=indexing
                      tunnel: u8 33 -> [w204]
                      i -> [w205]
                      n225 = To Unsigned Byte Integer(number=w205) -> (unsigned 8bit integer=w202:u8)
                      n226 = Add(x=w204, y=w202) -> (x+y=w203:u8)
                      n227 = call "write to RF synth bd.vi"("Address Byte"=w203, "BD 2 Byte"=w206, "BD 1 Byte"=w207) -> ()
                    }
                  }
                }
              }
            }
          }
        }
      }
    }
  }
  n228 = disable-structure shown="Disabled" {
    disable-tunnel: w2 -> [w448 _]
    frame Disabled {
      n229 = while "Excitation laser intensity feedback measurement (all lasers)" {
        shift-right: [w449] -> _
        shift-left: w448 -> [w454]
        stop <- FALSE stop-if-true
        n230 = flat-sequence {
          tunnel: w454 -> [w456]
          tunnel: [w457] -> w452
          tunnel: [w456] -> w450
          tunnel: [w463] -> w453
          tunnel: w452 -> [w463]
          tunnel: [w462] -> w451
          tunnel: w450 -> [w462]
          tunnel: [w475] -> w449
          tunnel: w453 -> [w486]
          tunnel: w451 -> [w483]
          frame #0 {
            n231 = call "Loop Timer9"("Count(Ticks)"=w456) -> ("Tick Count(Ticks)"=w457:u16)
          }
          frame #1 {
            # "Design note:\n\nAll lasers need to be measured at the same \ntime because the AI expansion module\ncannot independently time the measurements\nwithin our requirements: their is dead time.\n\nThis probably wouldn't be an issue with the built\nin AI on the fpga board itself."
            n232 = xnode "FPGA I/O Node"("Connector1/DIO35"=TRUE) -> ("Chassis2/Mod2/AI2"=→"Blue Intensity":i16, "Chassis2/Mod2/AI1"=→"Red FB Intensity":i16, "Chassis2/Mod2/AI0"=→"Green FB Sum":i16)  [unwired: 4 in, 4 out]
          }
          frame #2 {
            n233 = feedback-in #16(w486) -> ()
            n234 = feedback #16(w486) -> (w485:u16)
            n235 = Subtract(x=w486, y=w485) -> (x-y=w484:u16)
            n236 = xnode "FPGA I/O Node"("Connector1/DIO35"=FALSE) -> ()  [unwired: 1 in, 1 out]
            n237 = Subtract(x=w484, y=w483) -> (x-y=w465:u16)
            n238 = Subtract(x="Green FB Count", y=w465) -> (x-y=w479:u16)
            n239 = Number To Boolean Array(number=w465) -> (Boolean array=w466:bool[])
            n240 = Or Array Elements(Boolean array=w466) -> (logical OR=w464:bool)
            n241 = Boolean To (0,1)(Boolean="+ phase (Green FB)") -> (0, 1=w477:i16)
            n242 = Boolean To (0,1)(Boolean=w464) -> (0, 1=w471:i16)
            n243 = Multiply(x=w477, y="Phase count adjustment (Green FB)") -> (x*y=w472:i16)
            n244 = Add(x=w479, y=w472) -> (x+y=w475:u16)
            n245 = To Unsigned Byte Integer(number=w471) -> (unsigned 8bit integer=w468:u8)
            n246 = feedback #17(i16 0) -> (w474:i16)
            n247 = Subtract(x=w474, y=w472) -> (x-y=w473:i16)
            "Green FB Relative Phase" <- w473
            n248 = feedback-in #17(w473) -> ()
            n249 = feedback #18(u8 0) -> (w469:u8)
            n250 = Add(x=w468, y=w469) -> (x+y=w467:u8)
            "Green Late Counter" <- w467
            n251 = feedback-in #18(w467) -> ()
          }
        }
      }
    }
    frame Enabled {
    }
  }
  n252 = while "RF box board direct communication loop" {
    tunnel: w2 -> [_]
    stop <- FALSE stop-if-true
    n253 = case "Whether to use direct communication method (only use one method at a time)" shown="True" "Direct RF Box \nCommunication" {
      frame False {
      }
      frame True {
        n254 = case shown="True" "Update Data" {
          frame False {
          }
          frame True {
            n255 = flat-sequence {
              frame #0 {
                n256 = First Call?() -> (First Call?: T/F=w490:bool)
                n257 = case shown="True" w490 {
                  frame False {
                  }
                  frame True {
                    # "If first time data updated, be sure to set WR high\nbefore setting data and address bits."
                    n258 = flat-sequence {
                      frame #0 {
                        n259 = xnode "FPGA I/O Node"("Connector1/DIO15"=TRUE) -> ()  [unwired: 1 in, 1 out]
                      }
                      frame #1 {
                        n260 = call "Wait"("Count(Ticks)"=u8 40 ("DO Delay 3 (Ticks)")) -> ()  [unwired: 1 out]
                      }
                    }
                  }
                }
              }
              frame #1 {
                n261 = Number To Boolean Array(number="Address") -> (Boolean array=w539:bool[])
                n262 = Number To Boolean Array(number="Data BD 1") -> (Boolean array=w540:bool[])
                n263 = Number To Boolean Array(number="Data BD 2") -> (Boolean array=w509:bool[])
                n264 = Index Array(array=w540, index=7) -> (element=w524:bool)
                n265 = Index Array(array=w540, index=6) -> (element=w523:bool)
                n266 = Index Array(array=w540, index=5) -> (element=w522:bool)
                n267 = Index Array(array=w540, index=4) -> (element=w521:bool)
                n268 = Index Array(array=w540, index=3) -> (element=w520:bool)
                n269 = Index Array(array=w540, index=2) -> (element=w519:bool)
                n270 = Index Array(array=w540, index=1) -> (element=w518:bool)
                n271 = Index Array(array=w540, index=0) -> (element=w517:bool)
                n272 = Index Array(array=w539, index=5) -> (element=w516:bool)
                n273 = Index Array(array=w539, index=4) -> (element=w515:bool)
                n274 = Index Array(array=w539, index=3) -> (element=w514:bool)
                n275 = Index Array(array=w539, index=2) -> (element=w513:bool)
                n276 = Index Array(array=w539, index=1) -> (element=w512:bool)
                n277 = Index Array(array=w539, index=0) -> (element=w511:bool)
                n278 = Index Array(array=w509, index=7) -> (element=w500:bool)
                n279 = Index Array(array=w509, index=6) -> (element=w499:bool)
                n280 = Index Array(array=w509, index=5) -> (element=w498:bool)
                n281 = Index Array(array=w509, index=4) -> (element=w497:bool)
                n282 = Index Array(array=w509, index=3) -> (element=w496:bool)
                n283 = Index Array(array=w509, index=2) -> (element=w495:bool)
                n284 = Index Array(array=w509, index=1) -> (element=w494:bool)
                n285 = Index Array(array=w509, index=0) -> (element=w493:bool)
                n286 = xnode "FPGA I/O Node"("Connector1/DIO0"=w524, "Connector1/DIO1"=w523, "Connector1/DIO2"=w522, "Connector1/DIO3"=w521, "Connector1/DIO4"=w520, "Connector1/DIO5"=w519, "Connector1/DIO6"=w518, "Connector1/DIO7"=w517, "Connector1/DIO8"=w516, "Connector1/DIO9"=w515, "Connector1/DIO10"=w514, "Connector1/DIO11"=w513, "Connector1/DIO12"=w512, "Connector1/DIO13"=w511, "Connector1/DIO20"=w500, "Connector1/DIO21"=w499, "Connector1/DIO22"=w498, "Connector1/DIO23"=w497, "Connector1/DIO24"=w496, "Connector1/DIO25"=w495, "Connector1/DIO26"=w494, "Connector1/DIO27"=w493) -> ()  [unwired: 22 in, 22 out]
              }
              frame #2 {
                # "wait and then apply write signal"
                n287 = call "Wait2"("Count(Ticks)"=u8 40 ("DO Delay 1 (Ticks)")) -> ()  [unwired: 1 out]
              }
              frame #3 {
                # "sending bit low writes data to board buffer"
                n288 = xnode "FPGA I/O Node"("Connector1/DIO15"=FALSE) -> ()  [unwired: 1 in, 1 out]
              }
              frame #4 {
                # "wait then return write signal"
                n289 = call "Wait3"("Count(Ticks)"=u8 40 ("DO Delay 2 (Ticks)")) -> ()  [unwired: 1 out]
              }
              frame #5 {
                # "sending bit high makes ready to\nwrite more data"
                n290 = xnode "FPGA I/O Node"("Connector1/DIO15"=TRUE) -> ()  [unwired: 1 in, 1 out]
              }
            }
          }
        }
      }
    }
  }
  n291 = disable-structure shown="Disabled" {
    disable-tunnel: w6 -> [w548 _]
    disable-tunnel: w2 -> [w547 _]
    frame Disabled {
      n292 = while "APD 2 Gating" {
        shift-right: [w552] -> _
        shift-left: w547 -> [w557]
        shift-right: [w551] -> _
        shift-left: w548 -> [w549]
        stop <- FALSE stop-if-true
        n293 = flat-sequence {
          tunnel: w557 -> [w560]
          tunnel: [w561] -> w555
          tunnel: [w560] -> w553
          tunnel: [w559] -> w550
          tunnel: w549 -> [w559]
          tunnel: [w564] -> w556
          tunnel: w555 -> [w564]
          tunnel: [w563] -> w554
          tunnel: w553 -> [w563]
          tunnel: w550 -> [w562]
          tunnel: [w586] -> w552
          tunnel: w556 -> [w596]
          tunnel: w554 -> [w594]
          tunnel: [w565] -> w551
          frame #0 {
            n294 = call "Loop Timer8"("Count(Ticks)"=w560) -> ("Tick Count(Ticks)"=w561:u16)
          }
          frame #1 {
            # "Signal maybe then sent through \na transistor before APD"
            n295 = xnode "FPGA I/O Node"("Connector0/DIO8"=w562, "Connector0/DIO9"=w562, "Connector0/DIO10"=w562, "Connector0/DIO11"=w562) -> ()  [unwired: 4 in, 4 out]
            "APD2 int gate" <- w562
          }
          frame #2 {
            n296 = local read "APD Gate ON Count"() -> (w579:u16)
            n297 = local read "APD Gate OFF Count"() -> (w578:u16)
            n298 = feedback #19(TRUE) -> (w591:bool)
            n299 = feedback-in #20(w596) -> ()
            n300 = feedback #20(w596) -> (w580:u16)
            n301 = Not(x=w591) -> (.not. x?=w589:bool)
            n302 = feedback-in #19(w589) -> ()
            n303 = Subtract(x=w596, y=w580) -> (x-y=w595:u16)
            n304 = Select(t=w579, s=w589, f=w578) -> (s? t:f=w593:u16)
            n305 = Subtract(x=w595, y=w594) -> (x-y=w571:u16)
            n306 = Subtract(x=w593, y=w571) -> (x-y=w585:u16)
            n307 = Number To Boolean Array(number=w571) -> (Boolean array=w570:bool[])
            n308 = Or Array Elements(Boolean array=w570) -> (logical OR=w569:bool)
            n309 = Boolean To (0,1)(Boolean="+ phase (APD 2 Gate)") -> (0, 1=w583:i16)
            n310 = Multiply(x=w583, y="Phase count adjustment (APD 2 Gate)") -> (x*y=w581:i16)
            n311 = Boolean To (0,1)(Boolean=w569) -> (0, 1=w576:i16)
            n312 = Add(x=w585, y=w581) -> (x+y=w586:u16)
            n313 = To Unsigned Byte Integer(number=w576) -> (unsigned 8bit integer=w573:u8)
            n314 = feedback #21(i16 0) -> (w588:i16)
            n315 = Subtract(x=w588, y=w581) -> (x-y=w587:i16)
            "APD 2 Gate Relative Phase" <- w587
            n316 = feedback-in #21(w587) -> ()
            n317 = feedback #22(u8 0) -> (w574:u8)
            n318 = Add(x=w573, y=w574) -> (x+y=w572:u8)
            "APD 2 Gate Late Counter" <- w572
            n319 = feedback-in #22(w572) -> ()
            n320 = local read "APD Gate Operating Mode"() -> (w577:u8)
            n321 = case shown="2" w577 {
              tunnel: [TRUE FALSE w599] -> w566
              tunnel: w591 -> [_ _ w599]
              frame 0, Default {
              }
              frame 1 {
              }
              frame 2 {
              }
            }
            n322 = local read "Invert APD Gate"() -> (w568:bool)
            n323 = Not(x=w566) -> (.not. x?=w567:bool)
            n324 = Select(t=w567, s=w568, f=w566) -> (s? t:f=w565:bool)
          }
        }
      }
    }
    frame Enabled {
    }
  }
  n325 = disable-structure shown="Disabled" {
    disable-tunnel: w2 -> [w600 _]
    frame Disabled {
      n326 = while "APD 1 Counter" {
        tunnel: w600 -> [_]
        stop <- FALSE stop-if-true
        n327 = flat-sequence {
          frame #0 {
            n328 = xnode "FPGA I/O Method Node"("FPGA I/O In"=refnum<k21> "Connector0/DIO0" ("APD 1 DO"), "Timeout"=-1) -> ()  [unwired: 2 out]
          }
          frame #1 {
            n329 = local read "APD1 int gate"() -> (w604:bool)
            n330 = case shown="True" w604 {
              frame False {
              }
              frame True {
                n331 = local read "APD1 out state"() -> (w605:bool)
                n332 = case shown="True" w605 {
                  frame False {
                    n333 = local read "APD 1 Counts 0"() -> (w607:u32)
                    n334 = Increment(x=w607) -> (x+1=→"APD 1 Counts 0":u32)
                  }
                  frame True {
                    n335 = local read "APD 1 Counts 1"() -> (w609:u32)
                    n336 = Increment(x=w609) -> (x+1=→"APD 1 Counts 1":u32)
                  }
                }
              }
            }
          }
        }
      }
      n337 = while "APD 2 Counter" {
        tunnel: w600 -> [_]
        stop <- FALSE stop-if-true
        n338 = flat-sequence {
          frame #0 {
            n339 = xnode "FPGA I/O Method Node"("FPGA I/O In"=refnum<k21> "Connector0/DIO1" ("APD 2 DO"), "Timeout"=-1) -> ()  [unwired: 2 out]
          }
          frame #1 {
            n340 = local read "APD2 int gate"() -> (w613:bool)
            n341 = case shown="True" w613 {
              frame False {
              }
              frame True {
                n342 = local read "APD2 out state"() -> (w614:bool)
                n343 = case shown="False" w614 {
                  frame False {
                    n344 = local read "APD 2 Counts 0"() -> (w616:u32)
                    n345 = Increment(x=w616) -> (x+1=→"APD 2 Counts 0":u32)
                  }
                  frame True {
                    n346 = local read "APD 2 Counts 1"() -> (w618:u32)
                    n347 = Increment(x=w618) -> (x+1=→"APD 2 Counts 1":u32)
                  }
                }
              }
            }
          }
        }
      }
    }
    frame Enabled {
    }
  }
  n348 = disable-structure shown="Disabled" {
    disable-tunnel: w6 -> [w620 _]
    disable-tunnel: w2 -> [w619 _]
    frame Disabled {
      n349 = while "APD 1 Gating" {
        shift-right: [w624] -> _
        shift-left: w619 -> [w629]
        shift-right: [w623] -> _
        shift-left: w620 -> [w621]
        stop <- FALSE stop-if-true
        n350 = flat-sequence {
          tunnel: w629 -> [w632]
          tunnel: [w633] -> w627
          tunnel: [w632] -> w625
          tunnel: [w631] -> w622
          tunnel: w621 -> [w631]
          tunnel: [w636] -> w628
          tunnel: w627 -> [w636]
          tunnel: [w635] -> w626
          tunnel: w625 -> [w635]
          tunnel: w622 -> [w634]
          tunnel: [w654] -> w624
          tunnel: w628 -> [w668]
          tunnel: w626 -> [w665]
          tunnel: [w637] -> w623
          frame #0 {
            n351 = call "Loop Timer7"("Count(Ticks)"=w632) -> ("Tick Count(Ticks)"=w633:u16)
          }
          frame #1 {
            # "Signal maybe then sent through \na transistor before APD"
            n352 = xnode "FPGA I/O Node"("Connector0/DIO4"=w634, "Connector0/DIO5"=w634, "Connector0/DIO6"=w634, "Connector0/DIO7"=w634) -> ()  [unwired: 4 in, 4 out]
            "APD1 int gate" <- w634
          }
          frame #2 {
            n353 = feedback #23(TRUE) -> (w660:bool)
            n354 = feedback-in #24(w668) -> ()
            n355 = feedback #24(w668) -> (w667:u16)
            n356 = Not(x=w660) -> (.not. x?=w657:bool)
            n357 = feedback-in #23(w657) -> ()
            n358 = Subtract(x=w668, y=w667) -> (x-y=w666:u16)
            n359 = Select(t="APD Gate ON Count", s=w657, f="APD Gate OFF Count") -> (s? t:f=w662:u16)
            n360 = Subtract(x=w666, y=w665) -> (x-y=w642:u16)
            n361 = Subtract(x=w662, y=w642) -> (x-y=w653:u16)
            n362 = Number To Boolean Array(number=w642) -> (Boolean array=w643:bool[])
            n363 = Or Array Elements(Boolean array=w643) -> (logical OR=w641:bool)
            n364 = Boolean To (0,1)(Boolean="+ phase (APD 1 Gate)") -> (0, 1=w651:i16)
            n365 = Boolean To (0,1)(Boolean=w641) -> (0, 1=w648:i16)
            n366 = Multiply(x=w651, y="Phase count adjustment (APD 1 Gate)") -> (x*y=w649:i16)
            n367 = To Unsigned Byte Integer(number=w648) -> (unsigned 8bit integer=w645:u8)
            n368 = Add(x=w653, y=w649) -> (x+y=w654:u16)
            n369 = feedback #25(i16 0) -> (w656:i16)
            n370 = Subtract(x=w656, y=w649) -> (x-y=w655:i16)
            "APD 1 Gate Relative Phase" <- w655
            n371 = feedback-in #25(w655) -> ()
            n372 = feedback #26(u8 0) -> (w646:u8)
            n373 = Add(x=w645, y=w646) -> (x+y=w644:u8)
            "APD 1 Gate Late Counter" <- w644
            n374 = feedback-in #26(w644) -> ()
            n375 = case shown="2" "APD Gate Operating Mode" {
              tunnel: [TRUE FALSE w671] -> w638
              tunnel: w660 -> [_ _ w671]
              frame 0, Default {
              }
              frame 1 {
              }
              frame 2 {
              }
            }
            n376 = Not(x=w638) -> (.not. x?=w639:bool)
            n377 = Select(t=w639, s="Invert APD Gate", f=w638) -> (s? t:f=w637:bool)
          }
        }
      }
    }
    frame Enabled {
    }
  }
  n378 = disable-structure shown="Disabled" {
    disable-tunnel: u16 0 -> [w674 _]
    disable-tunnel: w4 -> [w673 _]
    disable-tunnel: w2 -> [w672 _]
    frame Disabled {
      n379 = while "532 nm green fluorescent laser interlacing (DO to IA 532 nm AOM ME amp)." {
        shift-right: [w789] -> _
        shift-left: w672 -> [w794]
        shift-right: [w788] -> _
        shift-left: w673 -> [w786]
        stop <- FALSE stop-if-true
        n380 = flat-sequence {
          tunnel: w794 -> [w797]
          tunnel: [w798] -> w792
          tunnel: [w797] -> w790
          tunnel: [w796] -> w787
          tunnel: w786 -> [w796]
          tunnel: [w801] -> w793
          tunnel: w792 -> [w801]
          tunnel: [w800] -> w791
          tunnel: w790 -> [w800]
          tunnel: w787 -> [w799]
          tunnel: [w810] -> w789
          tunnel: w793 -> [w830]
          tunnel: w791 -> [w827]
          tunnel: [w819] -> w788
          frame #0 {
            n381 = call "Loop Timer4"("Count(Ticks)"=w797) -> ("Tick Count(Ticks)"=w798:u16)
          }
          frame #1 {
            n382 = xnode "FPGA I/O Node"("Connector1/DIO34"=w799, "Connector1/DIO38"=w799, "Connector1/DIO39"=w799) -> ()  [unwired: 3 in, 3 out]
          }
          frame #2 {
            n383 = feedback-in #27(w830) -> ()
            n384 = feedback #27(w830) -> (w829:u16)
            n385 = Subtract(x=w830, y=w829) -> (x-y=w828:u16)
            n386 = Subtract(x=w828, y=w827) -> (x-y=w803:u16)
            n387 = Number To Boolean Array(number=w803) -> (Boolean array=w804:bool[])
            n388 = Or Array Elements(Boolean array=w804) -> (logical OR=w802:bool)
            n389 = Boolean To (0,1)(Boolean="+ phase (GI)") -> (0, 1=w815:i16)
            n390 = Multiply(x=w815, y="Phase count adjustment (GI)") -> (x*y=w812:i16)
            n391 = Boolean To (0,1)(Boolean=w802) -> (0, 1=w809:i16)
            n392 = To Unsigned Byte Integer(number=w809) -> (unsigned 8bit integer=w806:u8)
            n393 = feedback #28(i16 0) -> (w813:i16)
            n394 = feedback #29(u8 0) -> (w807:u8)
            n395 = Add(x=w806, y=w807) -> (x+y=w805:u8)
            "GI Late Counter" <- w805
            n396 = feedback-in #29(w805) -> ()
            n397 = Subtract(x=w813, y=w812) -> (x-y=w811:i16)
            "GI Relative phase" <- w811
            n398 = feedback-in #28(w811) -> ()
            n399 = feedback #30(TRUE) -> (w822:bool)
            n400 = case shown="2" "Operating Mode" {
              tunnel: [TRUE FALSE w836] -> w819
              tunnel: w822 -> [_ _ w833]
              frame 0, Default {
              }
              frame 1 {
              }
              frame 2 {
                n401 = Not(x=w833) -> (.not. x?=w835:bool)
                n402 = Select(t=w835, s="Invert GI", f=w833) -> (s? t:f=w836:bool)
              }
            }
            n403 = Not(x=w822) -> (.not. x?=w818:bool)
            n404 = Select(t="Green interlace ON count", s=w818, f="Green interlace OFF count") -> (s? t:f=w824:u16)
            n405 = Subtract(x=w824, y=w803) -> (x-y=w816:u16)
            n406 = Add(x=w816, y=w812) -> (x+y=w810:u16)
            n407 = feedback-in #30(w818) -> ()
          }
        }
      }
      n408 = while "Green and red fluorescent laser interlacing (Current AO to IA 532 nm AOM ME amp)." {
        shift-right: [w683] -> _
        shift-left: w672 -> [w686]
        shift-right: [w680] -> _
        shift-left: w674 -> [w678]
        shift-right: [w677] -> _
        shift-left: w674 -> [w676]
        stop <- FALSE stop-if-true
        n409 = flat-sequence {
          tunnel: w686 -> [w690]
          tunnel: [w691] -> w685
          tunnel: [w690] -> w684
          tunnel: [w689] -> w679
          tunnel: w678 -> [w689]
          tunnel: w676 -> [w688]
          tunnel: [w688] -> w675
          tunnel: [w695] -> w682
          tunnel: w685 -> [w695]
          tunnel: [w694] -> w681
          tunnel: w684 -> [w694]
          tunnel: w679 -> [w693]
          tunnel: w675 -> [w692]
          tunnel: [w708] -> w683
          tunnel: [w724] -> w680
          tunnel: w682 -> [w735]
          tunnel: w681 -> [w732]
          tunnel: [w698] -> w677
          frame #0 {
            n410 = call "Loop Timer10"("Count(Ticks)"=w690) -> ("Tick Count(Ticks)"=w691:u16)
          }
          frame #1 {
            n411 = xnode "FPGA I/O Node"("Chassis2/Mod1/AO0"=w693, "Chassis2/Mod1/AO1"=w692) -> ()  [unwired: 2 in, 2 out]
          }
          frame #2 {
            # "Design note:\n\nThese two laser controls are in the same loop\nbecause the expansion current AI cannot separately\ntime the outputs fast enough for us.  Apparently\nit is because of communication time between the\nexpansion card and the fpga.\n\nSo the two analog control signals have the same timing\nand profile, but independent amplitudes to independently\ncontrol the intensity and feedback for each laser."
            n412 = feedback #31(TRUE) -> (w696:bool)
            n413 = Not(x=w696) -> (.not. x?=w697:bool)
            n414 = feedback-in #31(w697) -> ()
            n415 = Subtract(x="Green interlace OFF count 2", y="Green int current ON count adj") -> (x-y=w717:u16)
            n416 = disable-structure shown="Disabled" {
              disable-tunnel: [w739 _] -> w698
              disable-tunnel: w696 -> [w736 _]
              frame Disabled {
                n417 = case shown="2" "RI Operating Mode 2" {
                  tunnel: [TRUE FALSE w751] -> w737
                  tunnel: w736 -> [_ _ w748]
                  frame 0, Default {
                  }
                  frame 1 {
                  }
                  frame 2 {
                    n418 = Not(x=w748) -> (.not. x?=w750:bool)
                    n419 = Select(t=w750, s="Invert RI 2", f=w748) -> (s? t:f=w751:bool)
                  }
                }
                n420 = And(x=w737, y="Red FB On/Off") -> (x .and. y?=w745:bool)
                n421 = case shown="True" w745 {
                  tunnel: "RI Current Out" -> [w752 _]
                  tunnel: [w752 w761] -> w741
                  frame False {
                  }
                  frame True {
                    n422 = local read "Red FB Intensity"() -> (w757:i16)
                    n423 = Bundle("P4"="P4", "I4"="I4", "D4"="D4") -> (w753:cluster{"P4":i16, "I4":i16, "D4":i16})  [unwired: 1 in]
                    n424 = call "Slower PID.vi"("process variable"=w757, "reset?"="Red FB Reset", "setpoint"="Red FB Setpoint", "PID gains (x 2^8)"=w753, "output range"=cluster{"output high":i16, "output low":i16} {"output high"=32767, "output low"=-32768} ("Green FB output range")) -> ("output"=w764:i16)  [unwired: 10 out]
                    n425 = To Long Integer(number=w764) -> (32bit integer=w758:i32)
                    n426 = Add(x=w758, y=32768) -> (x+y=w760:i32)
                    n427 = To Unsigned Word Integer(number=w760) -> (unsigned 16bit integer=w761:u16)
                  }
                }
                n428 = Boolean To (0,1)(Boolean=w737) -> (0, 1=w740:i16)
                n429 = To Unsigned Word Integer(number=w740) -> (unsigned 16bit integer=w742:u16)
                n430 = Multiply(x=w742, y=w741) -> (x*y=w739:u16)
              }
              frame Enabled {
              }
            }
            n431 = feedback-in #32(w735) -> ()
            n432 = feedback #32(w735) -> (w734:u16)
            n433 = Add(x="Green int current ON count adj", y="Green interlace ON count 2") -> (x+y=w718:u16)
            n434 = Subtract(x=w735, y=w734) -> (x-y=w733:u16)
            n435 = Select(t=w718, s=w697, f=w717) -> (s? t:f=w729:u16)
            n436 = Subtract(x=w733, y=w732) -> (x-y=w701:u16)
            n437 = Subtract(x=w729, y=w701) -> (x-y=w712:u16)
            n438 = case shown="2" "Operating Mode 2" {
              tunnel: [TRUE FALSE w785] -> w699
              tunnel: w696 -> [_ _ w782]
              frame 0, Default {
              }
              frame 1 {
              }
              frame 2 {
                n439 = Not(x=w782) -> (.not. x?=w784:bool)
                n440 = Select(t=w784, s="Invert GI 2", f=w782) -> (s? t:f=w785:bool)
              }
            }
            n441 = Number To Boolean Array(number=w701) -> (Boolean array=w702:bool[])
            n442 = Boolean To (0,1)(Boolean="+ phase (GI) 2") -> (0, 1=w714:i16)
            n443 = Or Array Elements(Boolean array=w702) -> (logical OR=w700:bool)
            n444 = Boolean To (0,1)(Boolean=w700) -> (0, 1=w707:i16)
            n445 = Multiply(x=w714, y="Phase count adjustment (GI) 2") -> (x*y=w710:i16)
            n446 = To Unsigned Byte Integer(number=w707) -> (unsigned 8bit integer=w703:u8)
            n447 = Add(x=w712, y=w710) -> (x+y=w708:u16)
            n448 = feedback #33(u8 0) -> (w705:u8)
            n449 = Add(x=w703, y=w705) -> (x+y=w704:u8)
            "GI Late Counter 2" <- w704
            n450 = feedback-in #33(w704) -> ()
            n451 = feedback #34(i16 0) -> (w711:i16)
            n452 = Subtract(x=w711, y=w710) -> (x-y=w709:i16)
            "GI Relative phase 2" <- w709
            n453 = feedback-in #34(w709) -> ()
            n454 = And(x=w699, y="Green FB On/Off") -> (x .and. y?=w719:bool)
            n455 = case shown="False" w719 {
              tunnel: "Current Out" -> [w766 _]
              tunnel: [w766 w775] -> w723
              frame False {
              }
              frame True {
                n456 = local read "Green FB Sum"() -> (w771:i16)
                n457 = Bundle("P3"="P3", "I3"="I3", "D3"="D3") -> (w767:cluster{"P3":i16, "I3":i16, "D3":i16})  [unwired: 1 in]
                n458 = call "Slower PID.vi"("process variable"=w771, "reset?"="Green FB Reset", "setpoint"="Green FB Setpoint", "PID gains (x 2^8)"=w767, "output range"=cluster{"output high":i16, "output low":i16} {"output high"=32767, "output low"=-32768} ("Green FB output range")) -> ("output"=w778:i16)  [unwired: 10 out]
                n459 = To Long Integer(number=w778) -> (32bit integer=w772:i32)
                n460 = Add(x=w772, y=32768) -> (x+y=w774:i32)
                n461 = To Unsigned Word Integer(number=w774) -> (unsigned 16bit integer=w775:u16)
              }
            }
            n462 = Boolean To (0,1)(Boolean=w699) -> (0, 1=w725:i16)
            n463 = To Unsigned Word Integer(number=w725) -> (unsigned 16bit integer=w722:u16)
            n464 = Multiply(x=w722, y=w723) -> (x*y=w724:u16)
          }
        }
      }
    }
    frame Enabled {
    }
  }
  n465 = while "MCL stage control" {
    shift-right: [w860] -> _
    shift-left: w2 -> [w863]
    shift-right: [w853] -> _
    shift-left: w11 -> [w850]
    shift-right: [w852] -> _
    shift-left: w10 -> [w848]
    shift-right: [w845] -> _
    shift-left: w1 -> [w841]
    shift-right: [w844] -> _
    shift-left: w1 -> [w839]
    shift-right: [w843] -> _
    shift-left: w1 -> [w837]
    stop <- FALSE stop-if-true
    n466 = flat-sequence {
      tunnel: w863 -> [w870]
      tunnel: [w871] -> w859
      tunnel: [w870] -> w857
      tunnel: [w869] -> w851
      tunnel: w850 -> [w869]
      tunnel: [w868] -> w849
      tunnel: w848 -> [w868]
      tunnel: [w867] -> w842
      tunnel: w841 -> [w867]
      tunnel: [w866] -> w840
      tunnel: w839 -> [w866]
      tunnel: [w865] -> w838
      tunnel: w837 -> [w865]
      tunnel: w859 -> [w878]
      tunnel: [w878] -> w858
      tunnel: w857 -> [w877]
      tunnel: [w877] -> w856
      tunnel: w851 -> [w876]
      tunnel: w849 -> [w875]
      tunnel: w842 -> [w874]
      tunnel: w840 -> [w873]
      tunnel: w838 -> [w872]
      tunnel: w858 -> [w891]
      tunnel: w856 -> [w890]
      tunnel: [w891] -> w862
      tunnel: [w890] -> w861
      tunnel: [w889] -> w855
      tunnel: [w888] -> w854
      tunnel: [w881] -> w847
      tunnel: [w879] -> w846
      tunnel: [w982] -> w860
      tunnel: w862 -> [w989]
      tunnel: w861 -> [w986]
      tunnel: w855 -> [w984]
      tunnel: w854 -> [w983]
      tunnel: [w984] -> w853
      tunnel: [w983] -> w852
      tunnel: w847 -> [w965]
      tunnel: w846 -> [w964]
      tunnel: ["Piezo Trap ON/Off (AO3)"] -> w845
      tunnel: [w965] -> w844
      tunnel: [w964] -> w843
      frame #0 {
        n467 = call "Loop Timer5"("Count(Ticks)"=w870) -> ("Tick Count(Ticks)"=w871:u32)
      }
      frame #1 {
        n468 = xnode "FPGA I/O Node"("Connector0/AO1"=w876, "Connector0/AO2"=w875, "Connector0/AO3"=w874, "Connector0/AO4"=w873, "Connector0/AO5"=w872) -> ()  [unwired: 5 in, 5 out]
      }
      frame #2 {
        n469 = local read "Scanning MCL"() -> (w903:bool)
        n470 = Or(x=w903, y="Start scan (MCL)") -> (x .or. y?=w898:bool)
        n471 = Not(x="Abort scan (MCL)") -> (.not. x?=w896:bool)
        n472 = And(x=w896, y=w898) -> (x .and. y?=w895:bool)
        n473 = case "Raster scan" shown="False" w895 {
          tunnel: [w920 w963] -> w900
          tunnel: "Start scan (MCL)" -> [_ w948]
          tunnel: [w920 w924] -> w884
          frame False {
            w920 = i16 0
            n474 = local write "Scanning MCL"(FALSE ("scanning")) -> ()
          }
          frame True {
            w934 = i16 0
            w933 = u64 0
            # "scan incr."
            # "freq. incr. mult."
            # "count steps"
            # "count number of cycles"
            n475 = feedback #35(w933) -> (w960:u64)
            n476 = Select(t=w933, s=w948, f=w960) -> (s? t:f=w962:u64)
            n477 = Increment(x=w962) -> (x+1=w959:u64)
            n478 = Greater?(x="Cycles per step (MCL)", y=w959) -> (0:w943:bool)
            n479 = Select(t=w959, s=w943, f=w933) -> (s? t:f=w958:u64)
            n480 = feedback-in #35(w958) -> ()
            n481 = feedback #36(w933) -> (w957:u64)
            n482 = Select(t=w933, s=w948, f=w957) -> (s? t:f=w952:u64)
            n483 = Increment(x=w952) -> (x+1=w956:u64)
            n484 = Add(x="Scan steps (MCL)", y="Scan steps (MCL)") -> (x+y=w955:u64)
            n485 = Select(t=w952, s=w943, f=w956) -> (s? t:f=w938:u64)
            n486 = Greater?(x=w955, y=w938) -> (0:w937:bool)
            n487 = Select(t=w938, s=w937, f=w933) -> (s? t:f=w953:u64)
            n488 = feedback-in #36(w953) -> ()
            n489 = Equal?(x="Scan steps (MCL)", y=w938) -> (x = y?=w942:bool)
            n490 = Greater?(x="Scan steps (MCL)", y=w952) -> (0:w951:bool)
            n491 = feedback #37(w934) -> (w954:i16)
            n492 = Select(t=w934, s=w948, f=w954) -> (s? t:f=w940:i16)
            n493 = Increment(x=w940) -> (x+1=w950:i16)
            n494 = Decrement(x=w940) -> (x-1=w949:i16)
            n495 = Select(t=w950, s=w951, f=w949) -> (s? t:f=w941:i16)
            n496 = Select(t=w940, s=w942, f=w941) -> (s? t:f=w939:i16)
            n497 = Select(t=w940, s=w943, f=w939) -> (s? t:f=w935:i16)
            n498 = Select(t=w935, s=w937, f=w934) -> (s? t:f=w936:i16)
            n499 = feedback-in #37(w936) -> ()
            n500 = feedback #38(w933) -> (w947:u64)
            n501 = Select(t=w933, s=w948, f=w947) -> (s? t:f=w922:u64)
            n502 = Increment(x=w922) -> (x+1=w944:u64)
            n503 = Select(t=w922, s=w937, f=w944) -> (s? t:f=w923:u64)
            n504 = Greater?(x="Number of scans (MCL)", y=w923) -> (0:w930:bool)
            n505 = Multiply(x="Scan freq.  increment (MCL)", y=w940) -> (x*y=w963:i16)
            n506 = Select(t=TRUE, s="Cont. Scan (MCL)", f=w930) -> (s? t:f=w929:bool)
            "Scanning MCL" <- w929
            n507 = Select(t=w923, s=w929, f=w933) -> (s? t:f=w945:u64)
            n508 = feedback-in #38(w945) -> ()
            n509 = Increment(x=w923) -> (x+1=→"Scan I (MCL)":u64)
            n510 = To Word Integer(number=w922) -> (16bit integer=w925:i16)
            n511 = Multiply(x=w925, y="Scan freq.  increment (MCL)") -> (x*y=w924:i16)
          }
        }
        n512 = Select(t=w884, s="1D or 2D Scan?", f=i16 0) -> (s? t:f=w885:i16)
        n513 = Select(t=w900, s="MCL Scan Axis", f=w885) -> (s? t:f=w901:i16)
        n514 = Select(t=w885, s="MCL Scan Axis", f=w900) -> (s? t:f=w899:i16)
        n515 = case shown="False" "ScanTrap 3 or Fl-laser" {
          tunnel: w901 -> [w911 w913]
          tunnel: w899 -> [w910 w917]
          tunnel: "AO2 (X)" -> [w909 w918]
          tunnel: "AO1 (Y)" -> [w908 w919]
          tunnel: [w907 w919] -> w889
          tunnel: [w906 w918] -> w888
          tunnel: "Piezo Trap Y (AO4)" -> [w905 w914]
          tunnel: [w905 w912] -> w881
          tunnel: "Piezo Trap X (AO5)" -> [w904 w916]
          tunnel: [w904 w915] -> w879
          frame False {
            n516 = Add(x=w908, y=w911) -> (x+y=w907:i16)
            n517 = Add(x=w910, y=w909) -> (x+y=w906:i16)
          }
          frame True {
            n518 = Add(x=w914, y=w913) -> (x+y=w912:i16)
            n519 = Add(x=w916, y=w917) -> (x+y=w915:i16)
          }
        }
      }
      frame #3 {
        n520 = feedback-in #39(w989) -> ()
        n521 = feedback #39(w989) -> (w988:u32)
        n522 = Boolean To (0,1)(Boolean="+ phase (MCL)") -> (0, 1=w980:i16)
        n523 = Subtract(x=w989, y=w988) -> (x-y=w987:u32)
        n524 = Multiply(x=w980, y="Phase count adjustment (MCL)") -> (x*y=w976:i16)
        n525 = Subtract(x=w987, y=w986) -> (x-y=w968:u32)
        n526 = Subtract(x="MCL count", y=w968) -> (x-y=w978:u32)
        n527 = feedback #40(i16 0) -> (w977:i16)
        n528 = Subtract(x=w977, y=w976) -> (x-y=w975:i16)
        "MCL Relative Phase" <- w975
        n529 = feedback-in #40(w975) -> ()
        n530 = Number To Boolean Array(number=w968) -> (Boolean array=w969:bool[])
        n531 = Or Array Elements(Boolean array=w969) -> (logical OR=w967:bool)
        n532 = Boolean To (0,1)(Boolean=w967) -> (0, 1=w974:i16)
        n533 = Add(x=w978, y=w976) -> (x+y=w982:u32)
        n534 = To Unsigned Byte Integer(number=w974) -> (unsigned 8bit integer=w971:u8)
        n535 = feedback #41(u8 0) -> (w972:u8)
        n536 = Add(x=w971, y=w972) -> (x+y=w970:u8)
        "MCL Late Counter" <- w970
        n537 = feedback-in #41(w970) -> ()
        "Piezo Y out" <- w965
        "Piezo X out" <- w964
      }
    }
  }
  n538 = while "Control APD data integration - stream to host" {
    shift-right: [w994] -> _
    shift-left: w7 -> [w999]
    stop <- FALSE stop-if-true
    n539 = flat-sequence {
      tunnel: w999 -> [w1001]
      tunnel: [w1002] -> w997
      tunnel: [w1001] -> w995
      tunnel: [w1012] -> w998
      tunnel: w997 -> [w1012]
      tunnel: [w1011] -> w996
      tunnel: w995 -> [w1011]
      tunnel: [w1010] -> w993
      tunnel: [w1009] -> w992
      tunnel: [w1003] -> w991
      tunnel: [w1054] -> w994
      tunnel: w998 -> [w1064]
      tunnel: w996 -> [w1061]
      tunnel: w993 -> [w1047]
      tunnel: w992 -> [w1046]
      tunnel: w991 -> [w1034]
      frame #0 {
        n540 = call "Loop Timer6"("Count(Ticks)"=w1001) -> ("Tick Count(Ticks)"=w1002:u32)
      }
      frame #1 {
        n541 = flat-sequence {
          tunnel: [w1014] -> w1008
          tunnel: w1008 -> [w1017]
          tunnel: [w1021] -> w1007
          tunnel: [w1020] -> w1006
          tunnel: [w1017] -> w1005
          tunnel: [w1016] -> w1004
          tunnel: [w1028] -> w1009
          tunnel: [w1029] -> w1010
          tunnel: w1007 -> [w1029]
          tunnel: w1006 -> [w1028]
          tunnel: w1005 -> [w1027]
          tunnel: w1004 -> [w1026]
          tunnel: [w1026] -> w1003
          frame #0 {
            # "use separate variable so each APD won't\nhave to wait to read"
            n542 = feedback #42(FALSE) -> (w1013:bool)
            "APD1 out state" <- w1013
            "APD2 out state" <- w1013
            "APD3 out state" <- w1013
            n543 = Not(x=w1013) -> (.not. x?=w1014:bool)
            n544 = feedback-in #42(w1014) -> ()
          }
          frame #1 {
            n545 = local read "APD 3 Counts 1"() -> (w1019:u32)
            n546 = local read "APD 3 Counts 0"() -> (w1018:u32)
            n547 = local read "APD 1 Counts 1"() -> (w1025:u32)
            n548 = local read "APD 1 Counts 0"() -> (w1024:u32)
            n549 = local read "APD 2 Counts 1"() -> (w1023:u32)
            n550 = local read "APD 2 Counts 0"() -> (w1022:u32)
            n551 = Select(t=w1019, s=w1017, f=w1018) -> (s? t:f=w1016:u32)
            n552 = Select(t=w1025, s=w1017, f=w1024) -> (s? t:f=w1021:u32)
            n553 = Select(t=w1023, s=w1017, f=w1022) -> (s? t:f=w1020:u32)
          }
          frame #2 {
            n554 = case shown="False" w1027 {
              frame False {
                w1030 = u32 0 ("APD 1 Counts 0")
                n555 = local write "APD 1 Counts 0"(w1030) -> ()
                n556 = local write "APD 2 Counts 0"(w1030) -> ()
                n557 = local write "APD 3 Counts 0"(w1030) -> ()
              }
              frame True {
                w1031 = u32 0 ("APD 1 Counts 1")
                n558 = local write "APD 1 Counts 1"(w1031) -> ()
                n559 = local write "APD 2 Counts 1"(w1031) -> ()
                n560 = local write "APD 3 Counts 1"(w1031) -> ()
              }
            }
          }
        }
      }
      frame #2 {
        n561 = feedback-in #43(w1064) -> ()
        n562 = feedback #43(w1064) -> (w1063:u32)
        n563 = Subtract(x=w1064, y=w1063) -> (x-y=w1062:u32)
        n564 = Subtract(x=w1062, y=w1061) -> (x-y=w1039:u32)
        n565 = case shown="True" "APD to FIFO" {
          tunnel: w1047 -> [_ w1069]
          tunnel: w1046 -> [_ w1067]
          tunnel: w1034 -> [_ w1065]
          frame False {
          }
          frame True {
            n566 = flat-sequence {
              tunnel: 0 ("Timeout") -> [w1071]
              tunnel: w1069 -> [w1072]
              tunnel: [w1071] -> w1068
              tunnel: w1068 -> [w1073]
              tunnel: w1067 -> [w1074]
              tunnel: [w1073] -> w1066
              tunnel: w1066 -> [w1076]
              tunnel: w1065 -> [w1075]
              frame #0 {
                n567 = xnode ("FIFO Write")("Element"=w1072, "Timeout"=w1071) -> ()  [unwired: 1 in, 2 out]
              }
              frame #1 {
                n568 = xnode ("FIFO Write")("Element"=w1074, "Timeout"=w1073) -> ()  [unwired: 1 in, 2 out]
              }
              frame #2 {
                n569 = xnode ("FIFO Write")("Element"=w1075, "Timeout"=w1076) -> ()  [unwired: 1 in, 2 out]
              }
            }
          }
        }
        n570 = Subtract(x="APD Acq Rate Count", y=w1039) -> (x-y=w1055:u32)
        n571 = Number To Boolean Array(number=w1039) -> (Boolean array=w1040:bool[])
        n572 = Or Array Elements(Boolean array=w1040) -> (logical OR=w1038:bool)
        n573 = Boolean To (0,1)(Boolean=w1038) -> (0, 1=w1045:i16)
        n574 = To Unsigned Byte Integer(number=w1045) -> (unsigned 8bit integer=w1042:u8)
        n575 = feedback #44(u8 0) -> (w1043:u8)
        n576 = Add(x=w1042, y=w1043) -> (x+y=w1041:u8)
        "APD Acq Late Counter" <- w1041
        n577 = feedback-in #44(w1041) -> ()
        n578 = Boolean To (0,1)(Boolean="+ phase (APD Acq)") -> (0, 1=w1051:i16)
        n579 = Multiply(x=w1051, y="Phase Count Adjustment (APD Acq)") -> (x*y=w1048:i16)
        n580 = Add(x=w1055, y=w1048) -> (x+y=w1054:u32)
        n581 = feedback #45(i16 0) -> (w1053:i16)
        n582 = Subtract(x=w1053, y=w1048) -> (x-y=w1050:i16)
        "APD Acq Relative Phase" <- w1050
        n583 = feedback-in #45(w1050) -> ()
        n584 = To Word Integer(number=w1047) -> (16bit integer=w1056:i16)
        n585 = To Word Integer(number=w1034) -> (16bit integer=w1035:i16)
        n586 = To Word Integer(number=w1046) -> (16bit integer=w1057:i16)
        n587 = Multiply(x="APD AO scale factor", y=w1057) -> (x*y=w1036:i16)
        n588 = Multiply(x="APD AO scale factor", y=w1035) -> (x*y=w1032:i16)
        n589 = Multiply(x="APD AO scale factor", y=w1056) -> (x*y=w1037:i16)
        n590 = xnode "FPGA I/O Node"("Connector0/AO6"=w1037, "Connector0/AO7"=w1036, "Connector0/AO5"=w1032) -> ()  [unwired: 3 in, 3 out]
      }
    }
  }
  n591 = while "DAQ AI set 1" {
    shift-right: [w1077] -> _
    shift-left: w2 -> [w1082]
    stop <- FALSE stop-if-true
    n592 = flat-sequence {
      tunnel: w1082 -> [w1092]
      tunnel: [w1093] -> w1080
      tunnel: [w1092] -> w1079
      tunnel: [w1103] -> w1090
      tunnel: [w1102] -> w1089
      tunnel: [w1101] -> w1088
      tunnel: [w1100] -> w1087
      tunnel: [w1099] -> w1086
      tunnel: [w1098] -> w1085
      tunnel: [w1097] -> w1084
      tunnel: [w1096] -> w1083
      tunnel: [w1095] -> w1081
      tunnel: w1080 -> [w1095]
      tunnel: w1079 -> [w1094]
      tunnel: [w1094] -> w1078
      tunnel: [w1135] -> w1077
      tunnel: w1090 -> [w1161]
      tunnel: w1089 -> [w1127]
      tunnel: w1088 -> [w1128]
      tunnel: w1087 -> [w1108]
      tunnel: w1086 -> [w1151]
      tunnel: w1085 -> [w1150]
      tunnel: w1084 -> [w1149]
      tunnel: w1083 -> [w1148]
      tunnel: w1081 -> [w1145]
      tunnel: w1078 -> [w1142]
      frame #0 {
        n593 = call "Loop Timer3"("Count(Ticks)"=w1092) -> ("Tick Count(Ticks)"=w1093:u16)
      }
      frame #1 {
        n594 = xnode "FPGA I/O Node"("Connector1/DIO31"=TRUE ("Connector1/DIO33")) -> ("Connector0/AI0"=w1103:i16, "Connector0/AI1"=w1102:i16, "Connector0/AI2"=w1101:i16, "Connector0/AI3"=w1100:i16, "Connector0/AI4"=w1099:i16, "Connector0/AI5"=w1098:i16, "Connector0/AI6"=w1097:i16, "Connector0/AI7"=w1096:i16)  [unwired: 9 in, 9 out]
      }
      frame #2 {
        w1131 = FALSE ("AI to FIFO")
        # "Changed by Ronen - the X and Y values of the MCL trap are now sent to the trap position FIFO"
        # "Adjust phase after data acquired if button pressed"
        n595 = feedback #46(i16 1) -> (w1154:i16)
        n596 = Increment(x=w1154) -> (x+1=w1160:i16)
        n597 = Scale By Power Of 2(n="AI1 X Scale", x=w1127) -> (x*2^n=w1125:i16)
        n598 = Greater?(x=w1160, y="N of AI1 Int Acq Sets") -> (0:w1157:bool)
        n599 = Select(t=i16 1, s=w1157, f=w1160) -> (s? t:f=w1159:i16)
        n600 = feedback-in #46(w1159) -> ()
        n601 = Divide(x=w1125, y=w1108) -> (x/y=w1124:fxp<+/-,16,1>)
        n602 = feedback #47(w1131) -> (w1129:bool)
        n603 = feedback #48(w1131) -> (w1147:bool)
        n604 = case shown="1, Default" w1154 {
          tunnel: w1128 -> [w1186 w1193 _]
          tunnel: ["Set 1" "Set 2" "Set 3"] -> w1152
          tunnel: ["AI to FIFO" w1195 w1200] -> w1146
          tunnel: w1147 -> [_ w1195 w1200]
          tunnel: ["Trap Pos to FIFO" w1194 w1199] -> w1130
          tunnel: w1129 -> [_ w1194 w1199]
          tunnel: w1124 -> [w1185 w1192 _]
          tunnel: [w1184 w1190 FALSE] -> w1107
          tunnel: [w1183 w1191 u64 0 ("BD1 Frequency Out 2")] -> w1111
          frame 1, Default {
            n605 = local read "BD1 Frequency Out 1"() -> (w1183:u64)
            n606 = Compound Arithmetic op=AND("Trap Pos to FIFO", "Set 1", "AI to FIFO") -> (w1184:bool)
            "AI2 Y Sum Set 1" <- w1186
            "AI1 X Set 1" <- w1185
          }
          frame 2 {
            n607 = local read "BD1 Frequency Out 2"() -> (w1191:u64)
            n608 = Compound Arithmetic op=AND(w1194, "Set 2", w1195) -> (w1190:bool)
            "AI2 Y Sum Set 2" <- w1193
            "AI1 X Set 2" <- w1192
          }
          frame 3 {
          }
        }
        n609 = And(x=w1152, y=w1146) -> (x .and. y?=w1153:bool)
        n610 = case shown="True" w1153 {
          tunnel: w1161 -> [_ w1214]
          tunnel: w1127 -> [_ w1213]
          tunnel: w1128 -> [_ w1212]
          tunnel: w1108 -> [_ w1211]
          tunnel: w1151 -> [_ w1210]
          tunnel: w1150 -> [_ w1209]
          tunnel: w1149 -> [_ w1208]
          tunnel: w1148 -> [_ w1207]
          tunnel: 0 ("DMA buffer timeout") -> [_ w1216]
          frame False {
          }
          frame True {
            n611 = Build Array(w1214, w1213, w1212, w1211, w1210, w1209, w1208, w1207) -> (w1215:i16[])
            n612 = for {
              tunnel: w1215 -> [w1218] mode=indexing
              tunnel: w1216 -> [w1219]
              tunnel: [w1217] -> w1205 mode=indexing
              n613 = xnode ("FIFO Write")("Element"=w1218, "Timeout"=w1219) -> ("Timed Out?"=w1217:bool)  [unwired: 1 in, 1 out]
            }
            n614 = Or Array Elements(Boolean array=w1205) -> (logical OR=w1202:bool)
            n615 = Boolean To (0,1)(Boolean=w1202) -> (0, 1=w1204:i16)
            n616 = feedback #49(u16 0) -> (w1203:u16)
            n617 = Add(x=w1204, y=w1203) -> (x+y=w1201:u16)
            "Trap AI FIFO Timeout" <- w1201
            n618 = feedback-in #49(w1201) -> ()
          }
        }
        n619 = feedback-in #47(w1130) -> ()
        n620 = feedback-in #48(w1146) -> ()
        n621 = local read "Piezo Y out"() -> (w1105:i16)
        n622 = local read "Piezo X out"() -> (w1106:i16)
        n623 = case shown="True" w1107 {
          tunnel: w1111 -> [_ w1169]
          tunnel: [u8 0 w1166] -> w1110
          tunnel: w1106 -> [_ w1165]
          tunnel: w1105 -> [_ w1164]
          frame False {
          }
          frame True {
            n624 = Split Number(x=w1169) -> (hi(x)=w1170:u32, lo(x)=w1171:u32)
            n625 = Split Number(x=w1170) -> (lo(x)=w1172:u16)  [unwired: 1 out]
            n626 = Split Number(x=w1171) -> (hi(x)=w1173:u16, lo(x)=w1174:u16)
            n627 = Build Array "BD 1 nu Stack"(w1172, w1173, w1174, w1165, w1164) -> (w1168:u16[])
            n628 = for {
              tunnel: w1168 -> [w1181] mode=indexing
              shift-right: [w1177] -> w1166
              shift-left: u8 0 -> [w1178]
              n629 = xnode ("FIFO Method Node")("Element"=w1181, "Timeout"="Trap FIFO Set Timeout") -> ("Timed Out?"=w1180:bool)  [unwired: 1 in, 1 out]
              n630 = Boolean To (0,1)(Boolean=w1180) -> (0, 1=w1179:i16)
              n631 = To Unsigned Byte Integer(number=w1179) -> (unsigned 8bit integer=w1176:u8)
              n632 = Add(x=w1176, y=w1178) -> (x+y=w1177:u8)
            }
          }
        }
        n633 = To Unsigned Word Integer(number=w1110) -> (unsigned 16bit integer=w1109:u16)
        n634 = feedback #50(u16 0) -> (w1122:u16)
        n635 = Add(x=w1109, y=w1122) -> (x+y=w1121:u16)
        "Trap Pos FIFO Timeout" <- w1121
        n636 = feedback-in #50(w1121) -> ()
        n637 = feedback-in #51(w1145) -> ()
        n638 = feedback #51(w1145) -> (w1144:u16)
        n639 = Subtract(x=w1145, y=w1144) -> (x-y=w1143:u16)
        n640 = xnode "FPGA I/O Node"("Connector1/DIO31"=FALSE ("Connector1/DIO34")) -> ()  [unwired: 1 in, 1 out]
        n641 = Subtract(x=w1143, y=w1142) -> (x-y=w1113:u16)
        n642 = Boolean To (0,1)(Boolean="+ phase") -> (0, 1=w1138:i16)
        n643 = Multiply(x=w1138, y="Phase count adjustment") -> (x*y=w1132:i16)
        n644 = Subtract(x="ai count", y=w1113) -> (x-y=w1136:u16)
        n645 = Number To Boolean Array(number=w1113) -> (Boolean array=w1114:bool[])
        n646 = feedback #52(i16 0) -> (w1134:i16)
        n647 = Add(x=w1136, y=w1132) -> (x+y=w1135:u16)
        n648 = Subtract(x=w1134, y=w1132) -> (x-y=w1133:i16)
        "Relative phase" <- w1133
        n649 = feedback-in #52(w1133) -> ()
        n650 = Or Array Elements(Boolean array=w1114) -> (logical OR=w1112:bool)
        n651 = Boolean To (0,1)(Boolean=w1112) -> (0, 1=w1119:i16)
        n652 = To Unsigned Byte Integer(number=w1119) -> (unsigned 8bit integer=w1116:u8)
        n653 = feedback #53(u8 0) -> (w1117:u8)
        n654 = Add(x=w1116, y=w1117) -> (x+y=w1115:u8)
        "AI Late Counter" <- w1115
        n655 = feedback-in #53(w1115) -> ()
      }
    }
  }
  n656 = node-c288(w8) -> ()
  n657 = disable-structure shown="Disabled" {
    disable-tunnel: w2 -> [w1220 _]
    frame Disabled {
      n658 = while "APD 3 Counter" {
        tunnel: w1220 -> [_]
        stop <- FALSE stop-if-true
        n659 = flat-sequence {
          frame #0 {
            n660 = xnode "FPGA I/O Method Node"("FPGA I/O In"=refnum<k21> "Connector0/DIO2" ("APD 2 DO"), "Timeout"=-1) -> ()  [unwired: 2 out]
          }
          frame #1 {
            n661 = local read "APD3 int gate"() -> (w1224:bool)
            n662 = case shown="True" w1224 {
              frame False {
              }
              frame True {
                n663 = local read "APD3 out state"() -> (w1225:bool)
                n664 = case shown="True" w1225 {
                  frame False {
                    n665 = local read "APD 3 Counts 0"() -> (w1227:u32)
                    n666 = Increment(x=w1227) -> (x+1=→"APD 3 Counts 0":u32)
                  }
                  frame True {
                    n667 = local read "APD 3 Counts 1"() -> (w1229:u32)
                    n668 = Increment(x=w1229) -> (x+1=→"APD 3 Counts 1":u32)
                  }
                }
              }
            }
          }
        }
      }
    }
    frame Enabled {
    }
  }
  n669 = disable-structure shown="Disabled" {
    disable-tunnel: w6 -> [w1231 _]
    disable-tunnel: w2 -> [w1230 _]
    frame Disabled {
      n670 = while "APD 3 Gating" {
        shift-right: [w1235] -> _
        shift-left: w1230 -> [w1240]
        shift-right: [w1234] -> _
        shift-left: w1231 -> [w1232]
        stop <- FALSE stop-if-true
        n671 = flat-sequence {
          tunnel: w1240 -> [w1243]
          tunnel: [w1244] -> w1238
          tunnel: [w1243] -> w1236
          tunnel: [w1242] -> w1233
          tunnel: w1232 -> [w1242]
          tunnel: [w1247] -> w1239
          tunnel: w1238 -> [w1247]
          tunnel: [w1246] -> w1237
          tunnel: w1236 -> [w1246]
          tunnel: w1233 -> [w1245]
          tunnel: [w1268] -> w1235
          tunnel: w1239 -> [w1279]
          tunnel: w1237 -> [w1276]
          tunnel: [w1248] -> w1234
          frame #0 {
            n672 = call "Loop Timer15"("Count(Ticks)"=w1243) -> ("Tick Count(Ticks)"=w1244:u16)
          }
          frame #1 {
            # "Signal maybe then sent through \na transistor before APD"
            n673 = xnode "FPGA I/O Node"("Connector0/DIO12"=w1245, "Connector0/DIO13"=w1245, "Connector0/DIO14"=w1245, "Connector0/DIO15"=w1245) -> ()  [unwired: 4 in, 4 out]
            "APD3 int gate" <- w1245
          }
          frame #2 {
            n674 = local read "APD Gate OFF Count"() -> (w1253:u16)
            n675 = local read "APD Gate ON Count"() -> (w1254:u16)
            n676 = feedback #54(TRUE) -> (w1273:bool)
            n677 = feedback-in #55(w1279) -> ()
            n678 = feedback #55(w1279) -> (w1278:u16)
            n679 = Not(x=w1273) -> (.not. x?=w1271:bool)
            n680 = feedback-in #54(w1271) -> ()
            n681 = Subtract(x=w1279, y=w1278) -> (x-y=w1277:u16)
            n682 = Select(t=w1254, s=w1271, f=w1253) -> (s? t:f=w1275:u16)
            n683 = Subtract(x=w1277, y=w1276) -> (x-y=w1256:u16)
            n684 = Subtract(x=w1275, y=w1256) -> (x-y=w1267:u16)
            n685 = Number To Boolean Array(number=w1256) -> (Boolean array=w1257:bool[])
            n686 = Or Array Elements(Boolean array=w1257) -> (logical OR=w1255:bool)
            n687 = Boolean To (0,1)(Boolean=w1255) -> (0, 1=w1262:i16)
            n688 = Boolean To (0,1)(Boolean="+ phase (APD 3 Gate)") -> (0, 1=w1265:i16)
            n689 = To Unsigned Byte Integer(number=w1262) -> (unsigned 8bit integer=w1259:u8)
            n690 = Multiply(x=w1265, y="Phase count adjustment (APD 3 Gate)") -> (x*y=w1263:i16)
            n691 = feedback #56(u8 0) -> (w1260:u8)
            n692 = Add(x=w1259, y=w1260) -> (x+y=w1258:u8)
            "APD 3 Gate Late Counter" <- w1258
            n693 = feedback-in #56(w1258) -> ()
            n694 = Add(x=w1267, y=w1263) -> (x+y=w1268:u16)
            n695 = feedback #57(i16 0) -> (w1270:i16)
            n696 = Subtract(x=w1270, y=w1263) -> (x-y=w1269:i16)
            "APD 3 Gate Relative Phase" <- w1269
            n697 = feedback-in #57(w1269) -> ()
            n698 = local read "APD Gate Operating Mode"() -> (w1252:u8)
            n699 = case shown="2" w1252 {
              tunnel: [TRUE FALSE w1282] -> w1249
              tunnel: w1273 -> [_ _ w1282]
              frame 0, Default {
              }
              frame 1 {
              }
              frame 2 {
              }
            }
            n700 = local read "Invert APD Gate"() -> (w1251:bool)
            n701 = Not(x=w1249) -> (.not. x?=w1250:bool)
            n702 = Select(t=w1250, s=w1251, f=w1249) -> (s? t:f=w1248:bool)
          }
        }
      }
    }
    frame Enabled {
    }
  }
  n703 = disable-structure shown="Disabled" {
    disable-tunnel: w4 -> [w1284 _]
    disable-tunnel: w2 -> [w1283 _]
    frame Disabled {
      n704 = while "633 nm red  fluorescent laser interlacing (DO to IA 633 nm AOM ME amp)." {
        shift-right: [w1288] -> _
        shift-left: w1283 -> [w1293]
        shift-right: [w1287] -> _
        shift-left: w1284 -> [w1285]
        stop <- FALSE stop-if-true
        n705 = flat-sequence {
          tunnel: w1293 -> [w1296]
          tunnel: [w1297] -> w1291
          tunnel: [w1296] -> w1289
          tunnel: [w1295] -> w1286
          tunnel: w1285 -> [w1295]
          tunnel: [w1300] -> w1292
          tunnel: w1291 -> [w1300]
          tunnel: [w1299] -> w1290
          tunnel: w1289 -> [w1299]
          tunnel: w1286 -> [w1298]
          tunnel: [w1309] -> w1288
          tunnel: w1292 -> [w1329]
          tunnel: w1290 -> [w1326]
          tunnel: [w1318] -> w1287
          frame #0 {
            n706 = call "Loop Timer11"("Count(Ticks)"=w1296) -> ("Tick Count(Ticks)"=w1297:u16)
          }
          frame #1 {
            # "Then to PRL 440 amp"
            n707 = xnode "FPGA I/O Node"("Connector1/DIO32"=w1298) -> ()  [unwired: 1 in, 1 out]
          }
          frame #2 {
            n708 = feedback-in #58(w1329) -> ()
            n709 = feedback #58(w1329) -> (w1328:u16)
            n710 = Subtract(x=w1329, y=w1328) -> (x-y=w1327:u16)
            n711 = Subtract(x=w1327, y=w1326) -> (x-y=w1302:u16)
            n712 = Number To Boolean Array(number=w1302) -> (Boolean array=w1303:bool[])
            n713 = Or Array Elements(Boolean array=w1303) -> (logical OR=w1301:bool)
            n714 = Boolean To (0,1)(Boolean="+ phase (RI)") -> (0, 1=w1314:i16)
            n715 = Multiply(x=w1314, y="Phase count adjustment (RI)") -> (x*y=w1311:i16)
            n716 = Boolean To (0,1)(Boolean=w1301) -> (0, 1=w1308:i16)
            n717 = To Unsigned Byte Integer(number=w1308) -> (unsigned 8bit integer=w1305:u8)
            n718 = feedback #59(i16 0) -> (w1312:i16)
            n719 = feedback #60(u8 0) -> (w1306:u8)
            n720 = Add(x=w1305, y=w1306) -> (x+y=w1304:u8)
            "RI Late Counter" <- w1304
            n721 = feedback-in #60(w1304) -> ()
            n722 = Subtract(x=w1312, y=w1311) -> (x-y=w1310:i16)
            "RI Relative phase" <- w1310
            n723 = feedback-in #59(w1310) -> ()
            n724 = feedback #61(TRUE) -> (w1321:bool)
            n725 = case shown="2" "Red Laser Operating Mode" {
              tunnel: [TRUE FALSE w1335] -> w1318
              tunnel: w1321 -> [_ _ w1332]
              frame 0, Default {
              }
              frame 1 {
              }
              frame 2 {
                n726 = Not(x=w1332) -> (.not. x?=w1334:bool)
                n727 = Select(t=w1334, s="Invert RI", f=w1332) -> (s? t:f=w1335:bool)
              }
            }
            n728 = Not(x=w1321) -> (.not. x?=w1317:bool)
            n729 = Select(t="Red interlace ON count", s=w1317, f="Red interlace OFF count") -> (s? t:f=w1323:u16)
            n730 = Subtract(x=w1323, y=w1302) -> (x-y=w1315:u16)
            n731 = Add(x=w1315, y=w1311) -> (x+y=w1309:u16)
            n732 = feedback-in #61(w1317) -> ()
          }
        }
      }
    }
    frame Enabled {
    }
  }
  n733 = disable-structure shown="Disabled" {
    disable-tunnel: w2 -> [w1336 _]
    frame Disabled {
      n734 = while "Blue fluorescent laser interlacing (AO control direct to laser)." {
        shift-right: [w1343] -> _
        shift-left: w1336 -> [w1346]
        shift-right: [w1340] -> _
        shift-left: i16 0 -> [w1338]
        stop <- FALSE stop-if-true
        n735 = flat-sequence {
          tunnel: w1346 -> [w1349]
          tunnel: [w1350] -> w1345
          tunnel: [w1349] -> w1344
          tunnel: [w1348] -> w1339
          tunnel: w1338 -> [w1348]
          tunnel: [w1353] -> w1342
          tunnel: w1345 -> [w1353]
          tunnel: [w1352] -> w1341
          tunnel: w1344 -> [w1352]
          tunnel: w1339 -> [w1351]
          tunnel: [w1363] -> w1343
          tunnel: [w1379] -> w1340
          tunnel: w1342 -> [w1391]
          tunnel: w1341 -> [w1388]
          frame #0 {
            n736 = call "Loop Timer13"("Count(Ticks)"=w1349) -> ("Tick Count(Ticks)"=w1350:u16)
          }
          frame #1 {
            n737 = xnode "FPGA I/O Node"("Connector0/AO3"=w1351) -> ()  [unwired: 1 in, 1 out]
          }
          frame #2 {
            n738 = Subtract(x="Blue OFF count (AO)", y="Blue current ON count adj (AO)") -> (x-y=w1372:u16)
            n739 = feedback-in #62(w1391) -> ()
            n740 = feedback #62(w1391) -> (w1390:u16)
            n741 = Add(x="Blue current ON count adj (AO)", y="Blue ON count (AO)") -> (x+y=w1373:u16)
            n742 = Subtract(x=w1391, y=w1390) -> (x-y=w1389:u16)
            n743 = Subtract(x=w1389, y=w1388) -> (x-y=w1356:u16)
            n744 = Number To Boolean Array(number=w1356) -> (Boolean array=w1357:bool[])
            n745 = Boolean To (0,1)(Boolean="+ phase (BI AO)") -> (0, 1=w1369:i16)
            n746 = Or Array Elements(Boolean array=w1357) -> (logical OR=w1355:bool)
            n747 = Boolean To (0,1)(Boolean=w1355) -> (0, 1=w1362:i16)
            n748 = Multiply(x=w1369, y="Phase count adjustment (BI AO)") -> (x*y=w1365:i16)
            n749 = To Unsigned Byte Integer(number=w1362) -> (unsigned 8bit integer=w1358:u8)
            n750 = feedback #63(u8 0) -> (w1360:u8)
            n751 = Add(x=w1358, y=w1360) -> (x+y=w1359:u8)
            "BI Late Counter (AO)" <- w1359
            n752 = feedback-in #63(w1359) -> ()
            n753 = feedback #64(i16 0) -> (w1366:i16)
            n754 = Subtract(x=w1366, y=w1365) -> (x-y=w1364:i16)
            "BI Relative phase (AO)" <- w1364
            n755 = feedback-in #64(w1364) -> ()
            n756 = feedback #65(TRUE) -> (w1383:bool)
            n757 = case shown="2" "BI Operating Mode (AO)" {
              tunnel: [TRUE FALSE w1407] -> w1374
              tunnel: w1383 -> [_ _ w1404]
              frame 0, Default {
              }
              frame 1 {
              }
              frame 2 {
                n758 = Not(x=w1404) -> (.not. x?=w1406:bool)
                n759 = Select(t=w1406, s="Invert BI (AO)", f=w1404) -> (s? t:f=w1407:bool)
              }
            }
            n760 = And(x=w1374, y="Blue FB On/Off") -> (x .and. y?=w1375:bool)
            n761 = case shown="True" w1375 {
              tunnel: "BI Current Out" -> [w1392 _]
              tunnel: [w1392 w1394] -> w1378
              frame False {
              }
              frame True {
                n762 = local read "Blue Intensity"() -> (w1393:i16)
                n763 = Bundle("P5"="P5", "I5"="I5", "D5"="D5") -> (w1395:cluster{"P5":i16, "I5":i16, "D5":i16})  [unwired: 1 in]
                n764 = call "Slower PID.vi"("process variable"=w1393, "reset?"="Blue FB Reset", "setpoint"="Blue FB Setpoint", "PID gains (x 2^8)"=w1395, "output range"=cluster{"output high":i16, "output low":i16} {"output high"=32767, "output low"=0} ("Green FB output range")) -> ("output"=w1394:i16)  [unwired: 10 out]
              }
            }
            n765 = Not(x=w1383) -> (.not. x?=w1380:bool)
            n766 = Select(t=w1373, s=w1380, f=w1372) -> (s? t:f=w1385:u16)
            n767 = Subtract(x=w1385, y=w1356) -> (x-y=w1367:u16)
            n768 = Add(x=w1367, y=w1365) -> (x+y=w1363:u16)
            n769 = feedback-in #65(w1380) -> ()
            n770 = Boolean To (0,1)(Boolean=w1374) -> (0, 1=w1354:i16)
            n771 = Multiply(x=w1354, y=w1378) -> (x*y=w1379:i16)
          }
        }
      }
    }
    frame Enabled {
    }
  }
  n772 = disable-structure shown="Disabled" {
    disable-tunnel: w4 -> [w1409 _]
    disable-tunnel: w2 -> [w1408 _]
    frame Disabled {
      n773 = while "473 nm blue  fluorescent laser interlacing (DO to blue laser digital control input)." {
        shift-right: [w1413] -> _
        shift-left: w1408 -> [w1418]
        shift-right: [w1412] -> _
        shift-left: w1409 -> [w1410]
        stop <- FALSE stop-if-true
        n774 = flat-sequence {
          tunnel: w1418 -> [w1421]
          tunnel: [w1422] -> w1416
          tunnel: [w1421] -> w1414
          tunnel: [w1420] -> w1411
          tunnel: w1410 -> [w1420]
          tunnel: [w1425] -> w1417
          tunnel: w1416 -> [w1425]
          tunnel: [w1424] -> w1415
          tunnel: w1414 -> [w1424]
          tunnel: w1411 -> [w1423]
          tunnel: [w1434] -> w1413
          tunnel: w1417 -> [w1454]
          tunnel: w1415 -> [w1451]
          tunnel: [w1443] -> w1412
          frame #0 {
            n775 = call "Loop Timer14"("Count(Ticks)"=w1421) -> ("Tick Count(Ticks)"=w1422:u16)
          }
          frame #1 {
            n776 = xnode "FPGA I/O Node"("Connector1/DIO28"=w1423) -> ()  [unwired: 1 in, 1 out]
          }
          frame #2 {
            n777 = feedback-in #66(w1454) -> ()
            n778 = feedback #66(w1454) -> (w1453:u16)
            n779 = Subtract(x=w1454, y=w1453) -> (x-y=w1452:u16)
            n780 = Subtract(x=w1452, y=w1451) -> (x-y=w1427:u16)
            n781 = Number To Boolean Array(number=w1427) -> (Boolean array=w1428:bool[])
            n782 = Or Array Elements(Boolean array=w1428) -> (logical OR=w1426:bool)
            n783 = Boolean To (0,1)(Boolean="+ phase (BI D)") -> (0, 1=w1439:i16)
            n784 = Multiply(x=w1439, y="Phase count adjustment (BI D)") -> (x*y=w1436:i16)
            n785 = Boolean To (0,1)(Boolean=w1426) -> (0, 1=w1433:i16)
            n786 = To Unsigned Byte Integer(number=w1433) -> (unsigned 8bit integer=w1430:u8)
            n787 = feedback #67(i16 0) -> (w1437:i16)
            n788 = feedback #68(u8 0) -> (w1431:u8)
            n789 = Add(x=w1430, y=w1431) -> (x+y=w1429:u8)
            "Blue Late Counter (D)" <- w1429
            n790 = feedback-in #68(w1429) -> ()
            n791 = Subtract(x=w1437, y=w1436) -> (x-y=w1435:i16)
            "BI Relative phase (D)" <- w1435
            n792 = feedback-in #67(w1435) -> ()
            n793 = feedback #69(TRUE) -> (w1446:bool)
            n794 = case shown="2" "Blue Laser Operating Mode (D)" {
              tunnel: [TRUE FALSE w1460] -> w1443
              tunnel: w1446 -> [_ _ w1457]
              frame 0, Default {
              }
              frame 1 {
              }
              frame 2 {
                n795 = Not(x=w1457) -> (.not. x?=w1459:bool)
                n796 = Select(t=w1459, s="Invert BI (D)", f=w1457) -> (s? t:f=w1460:bool)
              }
            }
            n797 = Not(x=w1446) -> (.not. x?=w1442:bool)
            n798 = Select(t="Blue interlace ON count (D)", s=w1442, f="Blue interlace OFF count (D)") -> (s? t:f=w1448:u16)
            n799 = Subtract(x=w1448, y=w1427) -> (x-y=w1440:u16)
            n800 = Add(x=w1440, y=w1436) -> (x+y=w1434:u16)
            n801 = feedback-in #69(w1442) -> ()
          }
        }
      }
    }
    frame Enabled {
    }
  }
